vi "Checkers PvP.vi"() -> ()   [LabVIEW 2016]
uses:
  <vilib>/Utility/miscctls.llb/LVPositionTypeDef.ctl
  Game Info Global Variable.vi
  Board Layout Global Variable.vi
panel:
  out "P2 Bottom Right Marker":picture
  out "P2 Bottom Left Marker":picture
  out "P2 Top Left Marker":picture
  out "P2 Top Right Marker":picture
  out "P1 Bottom Left Marker":picture
  out "P1 Bottom Right Marker":picture
  out "P1 Top Right Marker":picture
  out "P1 Top Left Marker":picture
  in  "Save and Quit":bool
  out "Player 2 Name":string="Player 2"
  out "Player 1 Name":string="Player 1"
  out "P2 King 12":picture
  out "P2 King 11":picture
  out "P2 King 10":picture
  out "P2 King 9":picture
  out "P2 King 8":picture
  out "P2 King 7":picture
  out "P2 King 6":picture
  out "P2 King 5":picture
  out "P2 King 4":picture
  out "P2 King 3":picture
  out "P2 King 2":picture
  out "P2 King":picture
  out "P1 King 12":picture
  out "P1 King 11":picture
  out "P1 King 10":picture
  out "P1 King 9":picture
  out "P1 King 8":picture
  out "P1 King 7":picture
  out "P1 King 6":picture
  out "P1 King 5":picture
  out "P1 King 4":picture
  out "P1 King 3":picture
  out "P1 King 2":picture
  out "P1 King":picture
  out "P2 Piece Icon":picture
  out "P1 Piece Icon":picture
  out "P2 Piece 12":picture
  out "P2 Piece 11":picture
  out "P2 Piece 10":picture
  out "P2 Piece 9":picture
  out "P2 Piece 8":picture
  out "P2 Piece 7":picture
  out "P2 Piece 6":picture
  out "P2 Piece 5":picture
  out "P2 Piece 4":picture
  out "P2 Piece 3":picture
  out "P2 Piece 2":picture
  out "P1 Piece 12":picture caption="P1 Piece"
  out "P1 Piece 11":picture caption="P1 Piece"
  out "P1 Piece 10":picture caption="P1 Piece"
  out "P1 Piece 9":picture caption="P1 Piece"
  out "P1 Piece 8":picture caption="P1 Piece"
  out "P1 Piece 7":picture caption="P1 Piece"
  out "P1 Piece 6":picture caption="P1 Piece"
  out "P1 Piece 5":picture caption="P1 Piece"
  out "P1 Piece 4":picture caption="P1 Piece"
  out "P1 Piece 3":picture caption="P1 Piece"
  out "P2 Piece":picture
  out "P1 Piece 2":picture caption="P1 Piece"
  in  "TURN":bool
  out "Game String":string
  out "P2 Turn Light":bool
  out "P1 Turn Light":bool=TRUE
  out "P1 Piece":picture
  in  "stop":bool
  in  "Offer Draw":bool
  in  "Surrender":bool
  out "Player 2 Label":string="Player 1"
  out "Player 1 Label":string="Player 1"
  in  "Save":bool
  in  "Quit":bool
  # "Your Turn!"
  # "Your Turn!"
  # "678, \n56"
  # "764, \n56"
  # "512, \n56"
  # "594, \n56"
  # "637, \n99"
  # "469, \n99"
  # "553, \n99"
  # "720, \n99"
  # "355, \n141"
  # "400, \n141"
  # "512, \n140"
  # "594, \n140"
  # "678, \n140"
  # "828, \n141"
  # "873, \n141"
  # "764, \n140"
  # "828, \n184"
  # "873, \n184"
  # "355, \n184"
  # "400, \n184"
  # "469, \n183"
  # "553, \n183"
  # "637, \n183"
  # "720, \n183"
  # "355, \n225"
  # "828, \n225"
  # "873, \n225"
  # "400, \n225"
  # "764, \n224"
  # "512, \n224"
  # "595, \n224"
  # "678, \n224"
  # "828, \n267"
  # "873, \n267"
  # "355, \n267"
  # "400, \n267"
  # "469, \n266"
  # "553, \n266"
  # "720, \n266"
  # "637, \n266"
  # "355, \n309"
  # "828, \n309"
  # "400, \n309"
  # "873, \n309"
  # "678, \n308"
  # "764, \n308"
  # "512, \n308"
  # "595, \n308"
  # "355, \n351"
  # "400, \n351"
  # "873, \n351"
  # "828, \n351"
  # "553, \n350"
  # "637, \n350"
  # "720, \n350"
  # "469,\n350"
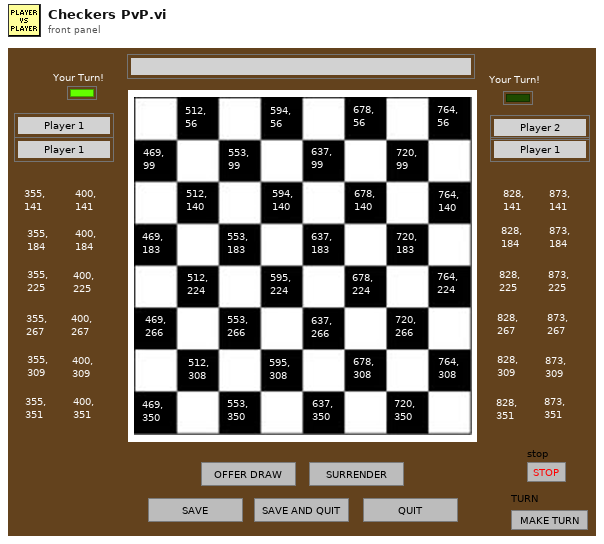
[diagram p1: front panel]
types:
  T1 = typedef "LVPositionTypeDef.ctl" = cluster{"Left":i32, "Top":i32}
  T2 = enum16{"Left Button", "Center Button", "Right Button", "Window Close"}
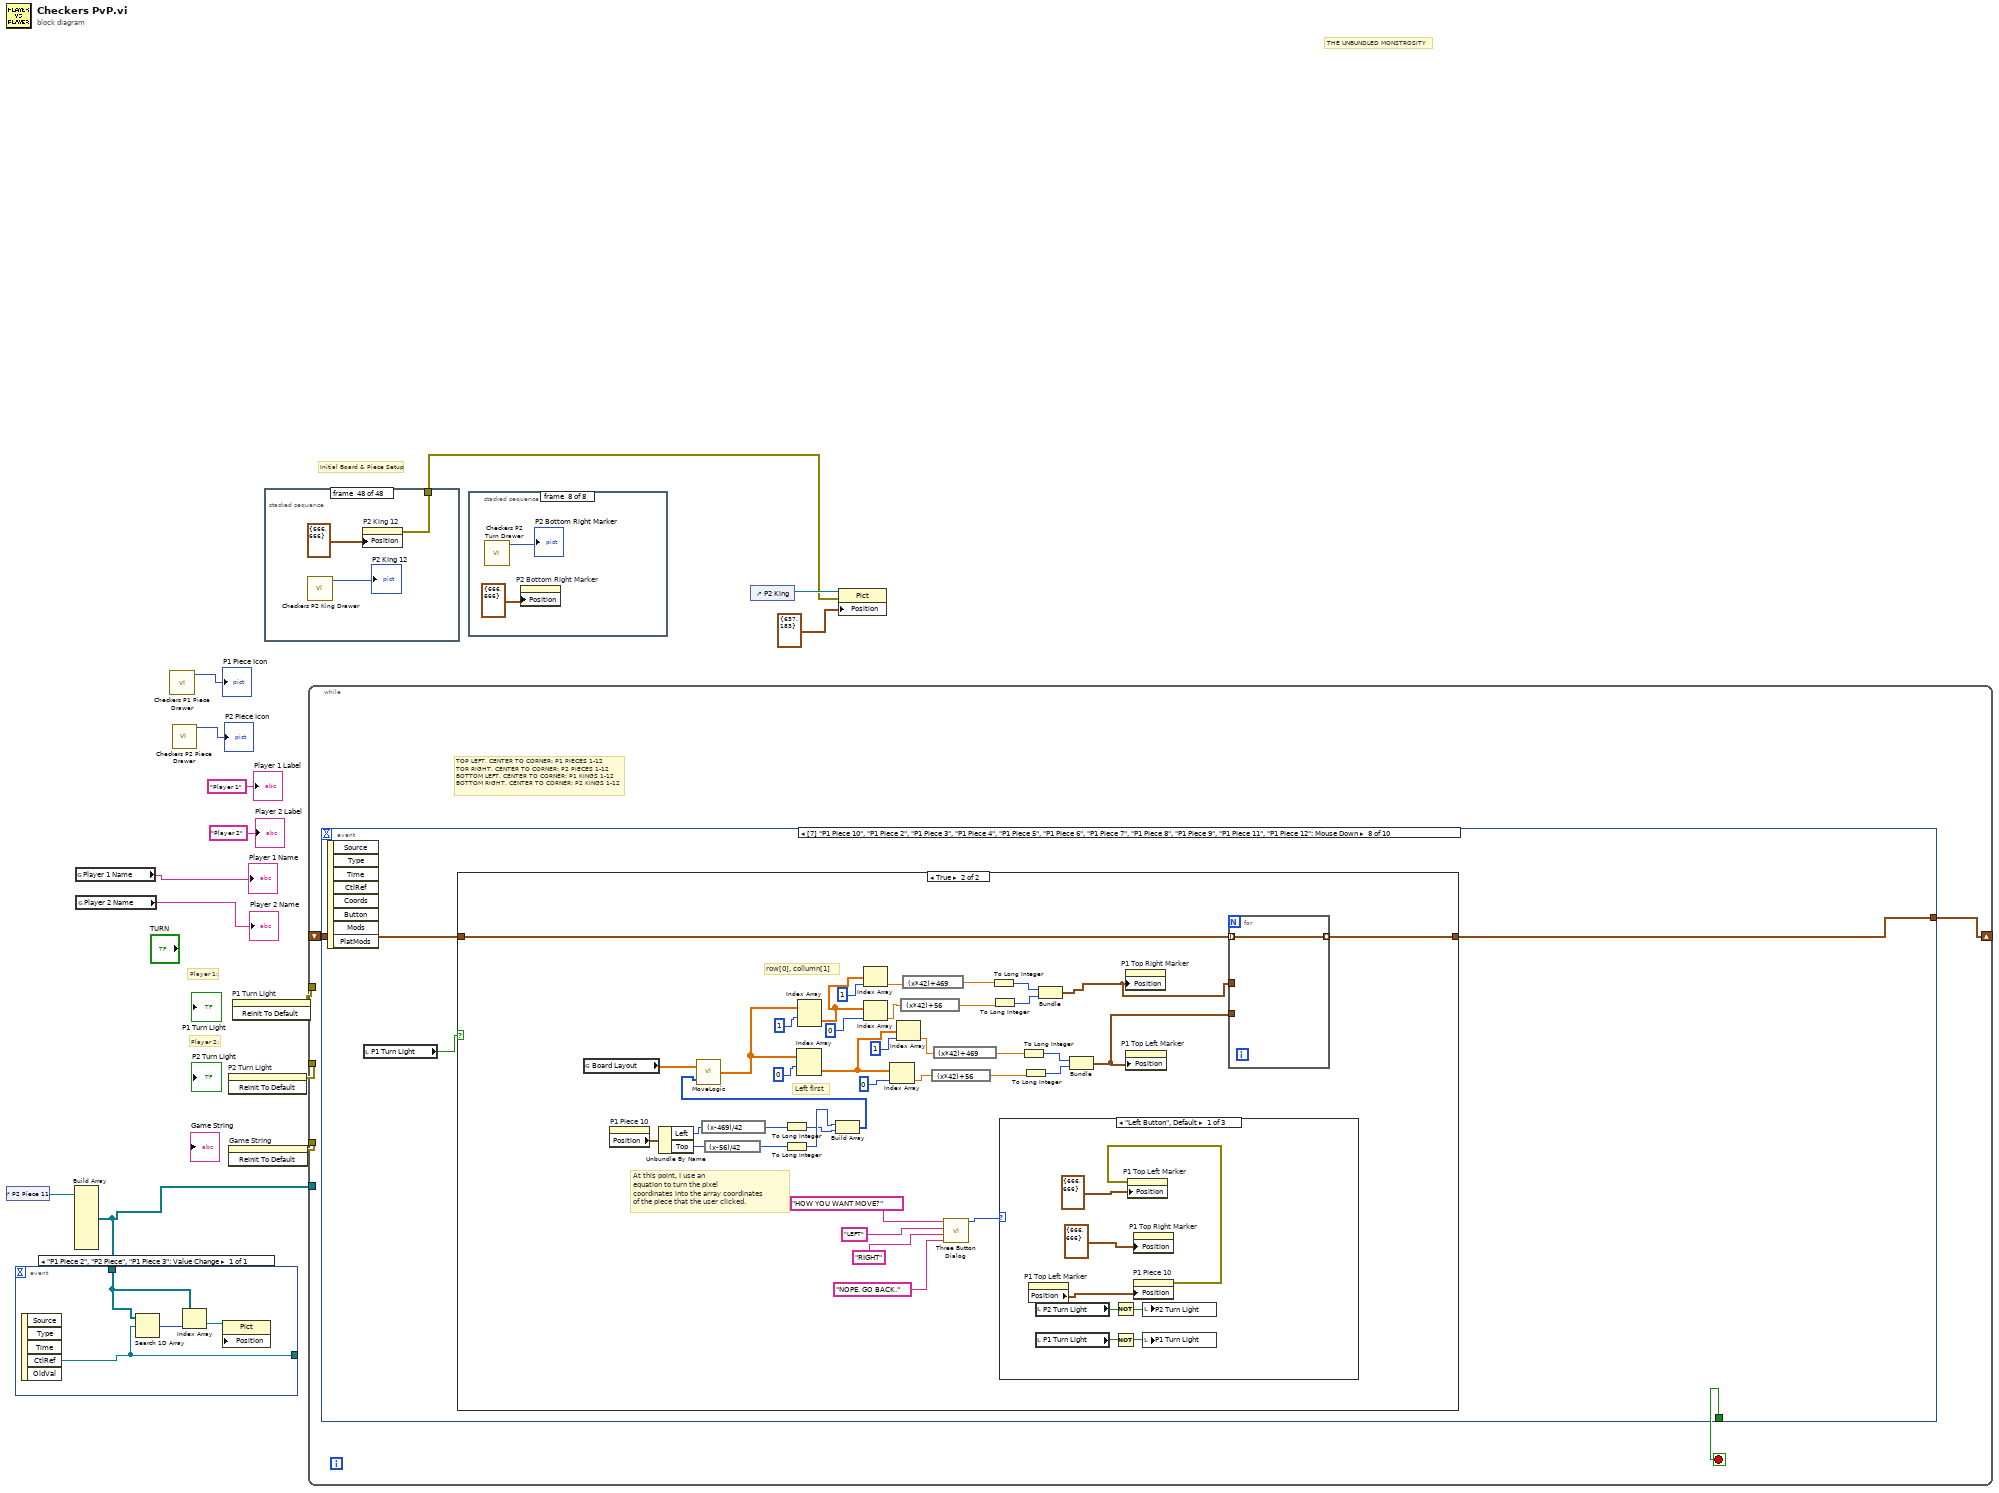
[diagram p0: block diagram]
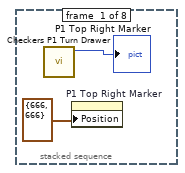
[diagram p2: hidden frame]
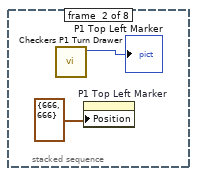
[diagram p3: hidden frame]
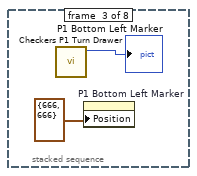
[diagram p4: hidden frame]
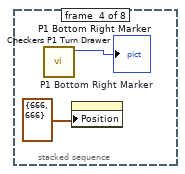
[diagram p5: hidden frame]
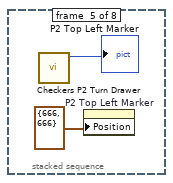
[diagram p6: hidden frame]
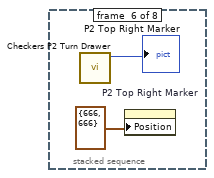
[diagram p7: hidden frame]
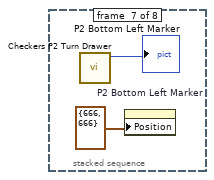
[diagram p8: hidden frame]
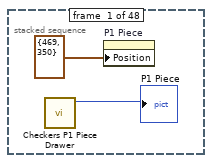
[diagram p9: hidden frame]
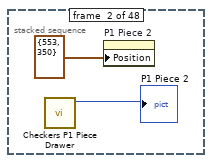
[diagram p10: hidden frame]
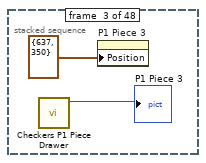
[diagram p11: hidden frame]
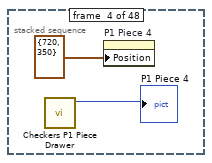
[diagram p12: hidden frame]
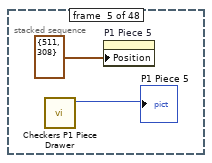
[diagram p13: hidden frame]
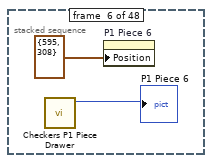
[diagram p14: hidden frame]
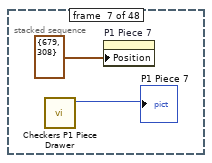
[diagram p15: hidden frame]
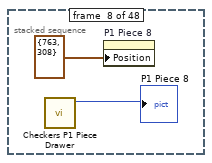
[diagram p16: hidden frame]
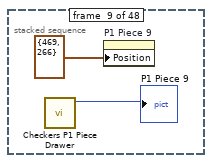
[diagram p17: hidden frame]
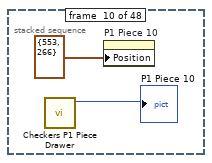
[diagram p18: hidden frame]
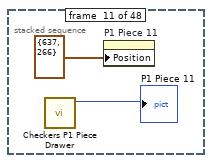
[diagram p19: hidden frame]
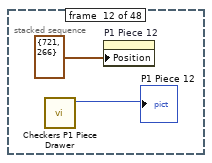
[diagram p20: hidden frame]
diagram:
  # "THE UNBUNDLED MONSTROSITY"
  # "Initial Board & Piece Setup"
  # "Player 2:"
  # "Player 1:"
  n1 = control-ref of="P2 Piece 11"() -> (w2:refnum<vi>)
  n2 = Build Array(w2) -> (w1:refnum<vi>[])  [unwired: 9 in]
  n3 = event shown="[0] \"P1 Piece 2\", \"P2 Piece\", \"P1 Piece 3\": Value Change" {
    selector: _ -> [_]
    dyn-events: _ -> [_]
    timeout: _ -> [_]
    tunnel: [w18] -> _
    tunnel: w1 -> [w17]
    event "P1 Piece 2", "P2 Piece", "P1 Piece 3": Value Change {
      n4 = event-data() -> ("CtlRef"=w18:refnum<vi>)  [unwired: 1 in, 4 out]
      n5 = Search 1D Array(1D array=w17, element=w18) -> (index of element=w16:i32)  [unwired: 1 in]
      n6 = Index Array(array=w17, index=w16) -> (element=w15:refnum<vi>)
      n7 = property class="Pict" props=["Position"](reference=w15) -> ()  [unwired: 2 in, 2 out]
    }
  }
  n8 = global read "Game Info Global Variable.vi" "Player 1 Name"() -> (→"Player 1 Name":string)
  n9 = global read "Game Info Global Variable.vi" "Player 2 Name"() -> (→"Player 2 Name":string)
  n10 = call "Checkers P1 Piece Drawer.vi"() -> ("new picture"=→"P1 Piece Icon":picture)  [unwired: 11 in]
  n11 = call "Checkers P2 Piece Drawer.vi"() -> ("new picture"=→"P2 Piece Icon":picture)  [unwired: 11 in]
  n12 = invoke on="P2 Turn Light" class="Bool (strict)" method="Reinit To Default"() -> (error out=w11:errorcluster)  [unwired: 3 in, 2 out]
  n13 = invoke on="Game String" class="Str" method="Reinit To Default"() -> (error out=w9:errorcluster)  [unwired: 3 in, 2 out]
  n14 = invoke on="P1 Turn Light" class="Bool (strict)" method="Reinit To Default"() -> (error out=w10:errorcluster)  [unwired: 3 in, 2 out]
  n15 = stacked-sequence {
    tunnel: [_ _ _ _ _ _ _ _ _ _ _ _ _ _ _ _ _ _ _ _ _ _ _ _ _ _ _ _ _ _ _ _ _ _ _ _ _ _ _ _ _ _ _ _ _ _ _ w113] -> w3
    frame #0 {
      n16 = call "Checkers P1 Piece Drawer.vi"() -> ("new picture"=→"P1 Piece":picture)  [unwired: 11 in]
      n17 = property on="P1 Piece" class="Pict"("Position"=T1 {"Left"=469, "Top"=350}) -> ()  [unwired: 2 in, 2 out]
    }
    frame #1 {
      n18 = call "Checkers P1 Piece Drawer.vi"() -> ("new picture"=→"P1 Piece 2":picture)  [unwired: 11 in]
      n19 = property on="P1 Piece 2" class="Pict"("Position"=T1 {"Left"=553, "Top"=350}) -> ()  [unwired: 2 in, 2 out]
    }
    frame #2 {
      n20 = call "Checkers P1 Piece Drawer.vi"() -> ("new picture"=→"P1 Piece 3":picture)  [unwired: 11 in]
      n21 = property on="P1 Piece 3" class="Pict"("Position"=T1 {"Left"=637, "Top"=350}) -> ()  [unwired: 2 in, 2 out]
    }
    frame #3 {
      n22 = call "Checkers P1 Piece Drawer.vi"() -> ("new picture"=→"P1 Piece 4":picture)  [unwired: 11 in]
      n23 = property on="P1 Piece 4" class="Pict"("Position"=T1 {"Left"=720, "Top"=350}) -> ()  [unwired: 2 in, 2 out]
    }
    frame #4 {
      n24 = call "Checkers P1 Piece Drawer.vi"() -> ("new picture"=→"P1 Piece 5":picture)  [unwired: 11 in]
      n25 = property on="P1 Piece 5" class="Pict"("Position"=T1 {"Left"=511, "Top"=308}) -> ()  [unwired: 2 in, 2 out]
    }
    frame #5 {
      n26 = call "Checkers P1 Piece Drawer.vi"() -> ("new picture"=→"P1 Piece 6":picture)  [unwired: 11 in]
      n27 = property on="P1 Piece 6" class="Pict"("Position"=T1 {"Left"=595, "Top"=308}) -> ()  [unwired: 2 in, 2 out]
    }
    frame #6 {
      n28 = call "Checkers P1 Piece Drawer.vi"() -> ("new picture"=→"P1 Piece 7":picture)  [unwired: 11 in]
      n29 = property on="P1 Piece 7" class="Pict"("Position"=T1 {"Left"=679, "Top"=308}) -> ()  [unwired: 2 in, 2 out]
    }
    frame #7 {
      n30 = call "Checkers P1 Piece Drawer.vi"() -> ("new picture"=→"P1 Piece 8":picture)  [unwired: 11 in]
      n31 = property on="P1 Piece 8" class="Pict"("Position"=T1 {"Left"=763, "Top"=308}) -> ()  [unwired: 2 in, 2 out]
    }
    frame #8 {
      n32 = call "Checkers P1 Piece Drawer.vi"() -> ("new picture"=→"P1 Piece 9":picture)  [unwired: 11 in]
      n33 = property on="P1 Piece 9" class="Pict"("Position"=T1 {"Left"=469, "Top"=266}) -> ()  [unwired: 2 in, 2 out]
    }
    frame #9 {
      n34 = call "Checkers P1 Piece Drawer.vi"() -> ("new picture"=→"P1 Piece 10":picture)  [unwired: 11 in]
      n35 = property on="P1 Piece 10" class="Pict"("Position"=T1 {"Left"=553, "Top"=266}) -> ()  [unwired: 2 in, 2 out]
    }
    frame #10 {
      n36 = call "Checkers P1 Piece Drawer.vi"() -> ("new picture"=→"P1 Piece 11":picture)  [unwired: 11 in]
      n37 = property on="P1 Piece 11" class="Pict"("Position"=T1 {"Left"=637, "Top"=266}) -> ()  [unwired: 2 in, 2 out]
    }
    frame #11 {
      n38 = call "Checkers P1 Piece Drawer.vi"() -> ("new picture"=→"P1 Piece 12":picture)  [unwired: 11 in]
      n39 = property on="P1 Piece 12" class="Pict"("Position"=T1 {"Left"=721, "Top"=266}) -> ()  [unwired: 2 in, 2 out]
    }
    frame #12 {
      n40 = call "Checkers P2 Piece Drawer.vi"() -> ("new picture"=→"P2 Piece":picture)  [unwired: 11 in]
      n41 = property on="P2 Piece" class="Pict"("Position"=T1 {"Left"=511, "Top"=140}) -> ()  [unwired: 2 in, 2 out]
    }
    frame #13 {
      n42 = call "Checkers P2 Piece Drawer.vi"() -> ("new picture"=→"P2 Piece 2":picture)  [unwired: 11 in]
      n43 = property on="P2 Piece 2" class="Pict"("Position"=T1 {"Left"=595, "Top"=140}) -> ()  [unwired: 2 in, 2 out]
    }
    frame #14 {
      n44 = call "Checkers P2 Piece Drawer.vi"() -> ("new picture"=→"P2 Piece 3":picture)  [unwired: 11 in]
      n45 = property on="P2 Piece 3" class="Pict"("Position"=T1 {"Left"=679, "Top"=140}) -> ()  [unwired: 2 in, 2 out]
    }
    frame #15 {
      n46 = call "Checkers P2 Piece Drawer.vi"() -> ("new picture"=→"P2 Piece 4":picture)  [unwired: 11 in]
      n47 = property on="P2 Piece 4" class="Pict"("Position"=T1 {"Left"=763, "Top"=140}) -> ()  [unwired: 2 in, 2 out]
    }
    frame #16 {
      n48 = call "Checkers P2 Piece Drawer.vi"() -> ("new picture"=→"P2 Piece 5":picture)  [unwired: 11 in]
      n49 = property on="P2 Piece 5" class="Pict"("Position"=T1 {"Left"=469, "Top"=98}) -> ()  [unwired: 2 in, 2 out]
    }
    frame #17 {
      n50 = call "Checkers P2 Piece Drawer.vi"() -> ("new picture"=→"P2 Piece 6":picture)  [unwired: 11 in]
      n51 = property on="P2 Piece 6" class="Pict"("Position"=T1 {"Left"=553, "Top"=98}) -> ()  [unwired: 2 in, 2 out]
    }
    frame #18 {
      n52 = call "Checkers P2 Piece Drawer.vi"() -> ("new picture"=→"P2 Piece 7":picture)  [unwired: 11 in]
      n53 = property on="P2 Piece 7" class="Pict"("Position"=T1 {"Left"=637, "Top"=98}) -> ()  [unwired: 2 in, 2 out]
    }
    frame #19 {
      n54 = call "Checkers P2 Piece Drawer.vi"() -> ("new picture"=→"P2 Piece 8":picture)  [unwired: 11 in]
      n55 = property on="P2 Piece 8" class="Pict"("Position"=T1 {"Left"=721, "Top"=98}) -> ()  [unwired: 2 in, 2 out]
    }
    frame #20 {
      n56 = call "Checkers P2 Piece Drawer.vi"() -> ("new picture"=→"P2 Piece 9":picture)  [unwired: 11 in]
      n57 = property on="P2 Piece 9" class="Pict"("Position"=T1 {"Left"=511, "Top"=56}) -> ()  [unwired: 2 in, 2 out]
    }
    frame #21 {
      n58 = call "Checkers P2 Piece Drawer.vi"() -> ("new picture"=→"P2 Piece 10":picture)  [unwired: 11 in]
      n59 = property on="P2 Piece 10" class="Pict"("Position"=T1 {"Left"=595, "Top"=56}) -> ()  [unwired: 2 in, 2 out]
    }
    frame #22 {
      n60 = call "Checkers P2 Piece Drawer.vi"() -> ("new picture"=→"P2 Piece 11":picture)  [unwired: 11 in]
      n61 = property on="P2 Piece 11" class="Pict"("Position"=T1 {"Left"=679, "Top"=56}) -> ()  [unwired: 2 in, 2 out]
    }
    frame #23 {
      n62 = call "Checkers P2 Piece Drawer.vi"() -> ("new picture"=→"P2 Piece 12":picture)  [unwired: 11 in]
      n63 = property on="P2 Piece 12" class="Pict"("Position"=T1 {"Left"=763, "Top"=56}) -> ()  [unwired: 2 in, 2 out]
    }
    frame #24 {
      n64 = call "Checkers P1 King Drawer.vi"() -> ("new picture"=→"P1 King":picture)  [unwired: 11 in]
      n65 = property on="P1 King" class="Pict"("Position"=T1 {"Left"=666, "Top"=666}) -> ()  [unwired: 2 in, 2 out]
    }
    frame #25 {
      n66 = call "Checkers P1 King Drawer.vi"() -> ("new picture"=→"P1 King 2":picture)  [unwired: 11 in]
      n67 = property on="P1 King 2" class="Pict"("Position"=T1 {"Left"=666, "Top"=666}) -> ()  [unwired: 2 in, 2 out]
    }
    frame #26 {
      n68 = call "Checkers P1 King Drawer.vi"() -> ("new picture"=→"P1 King 3":picture)  [unwired: 11 in]
      n69 = property on="P1 King 3" class="Pict"("Position"=T1 {"Left"=666, "Top"=666}) -> ()  [unwired: 2 in, 2 out]
    }
    frame #27 {
      n70 = call "Checkers P1 King Drawer.vi"() -> ("new picture"=→"P1 King 4":picture)  [unwired: 11 in]
      n71 = property on="P1 King 4" class="Pict"("Position"=T1 {"Left"=666, "Top"=666}) -> ()  [unwired: 2 in, 2 out]
    }
    frame #28 {
      n72 = call "Checkers P1 King Drawer.vi"() -> ("new picture"=→"P1 King 5":picture)  [unwired: 11 in]
      n73 = property on="P1 King 5" class="Pict"("Position"=T1 {"Left"=666, "Top"=666}) -> ()  [unwired: 2 in, 2 out]
    }
    frame #29 {
      n74 = call "Checkers P1 King Drawer.vi"() -> ("new picture"=→"P1 King 6":picture)  [unwired: 11 in]
      n75 = property on="P1 King 6" class="Pict"("Position"=T1 {"Left"=666, "Top"=666}) -> ()  [unwired: 2 in, 2 out]
    }
    frame #30 {
      n76 = call "Checkers P1 King Drawer.vi"() -> ("new picture"=→"P1 King 7":picture)  [unwired: 11 in]
      n77 = property on="P1 King 7" class="Pict"("Position"=T1 {"Left"=666, "Top"=666}) -> ()  [unwired: 2 in, 2 out]
    }
    frame #31 {
      n78 = call "Checkers P1 King Drawer.vi"() -> ("new picture"=→"P1 King 8":picture)  [unwired: 11 in]
      n79 = property on="P1 King 8" class="Pict"("Position"=T1 {"Left"=666, "Top"=666}) -> ()  [unwired: 2 in, 2 out]
    }
    frame #32 {
      n80 = call "Checkers P1 King Drawer.vi"() -> ("new picture"=→"P1 King 9":picture)  [unwired: 11 in]
      n81 = property on="P1 King 9" class="Pict"("Position"=T1 {"Left"=666, "Top"=666}) -> ()  [unwired: 2 in, 2 out]
    }
    frame #33 {
      n82 = call "Checkers P1 King Drawer.vi"() -> ("new picture"=→"P1 King 10":picture)  [unwired: 11 in]
      n83 = property on="P1 King 10" class="Pict"("Position"=T1 {"Left"=666, "Top"=666}) -> ()  [unwired: 2 in, 2 out]
    }
    frame #34 {
      n84 = call "Checkers P1 King Drawer.vi"() -> ("new picture"=→"P1 King 11":picture)  [unwired: 11 in]
      n85 = property on="P1 King 11" class="Pict"("Position"=T1 {"Left"=666, "Top"=666}) -> ()  [unwired: 2 in, 2 out]
    }
    frame #35 {
      n86 = call "Checkers P1 King Drawer.vi"() -> ("new picture"=→"P1 King 12":picture)  [unwired: 11 in]
      n87 = property on="P1 King 12" class="Pict"("Position"=T1 {"Left"=666, "Top"=666}) -> ()  [unwired: 2 in, 2 out]
    }
    frame #36 {
      n88 = call "Checkers P2 King Drawer.vi"() -> ("new picture"=→"P2 King":picture)  [unwired: 11 in]
      n89 = property on="P2 King" class="Pict"("Position"=T1 {"Left"=666, "Top"=666}) -> ()  [unwired: 2 in, 2 out]
    }
    frame #37 {
      n90 = call "Checkers P2 King Drawer.vi"() -> ("new picture"=→"P2 King 2":picture)  [unwired: 11 in]
      n91 = property on="P2 King 2" class="Pict"("Position"=T1 {"Left"=666, "Top"=666}) -> ()  [unwired: 2 in, 2 out]
    }
    frame #38 {
      n92 = call "Checkers P2 King Drawer.vi"() -> ("new picture"=→"P2 King 3":picture)  [unwired: 11 in]
      n93 = property on="P2 King 3" class="Pict"("Position"=T1 {"Left"=666, "Top"=666}) -> ()  [unwired: 2 in, 2 out]
    }
    frame #39 {
      n94 = call "Checkers P2 King Drawer.vi"() -> ("new picture"=→"P2 King 4":picture)  [unwired: 11 in]
      n95 = property on="P2 King 4" class="Pict"("Position"=T1 {"Left"=666, "Top"=666}) -> ()  [unwired: 2 in, 2 out]
    }
    frame #40 {
      n96 = call "Checkers P2 King Drawer.vi"() -> ("new picture"=→"P2 King 5":picture)  [unwired: 11 in]
      n97 = property on="P2 King 5" class="Pict"("Position"=T1 {"Left"=666, "Top"=666}) -> ()  [unwired: 2 in, 2 out]
    }
    frame #41 {
      n98 = call "Checkers P2 King Drawer.vi"() -> ("new picture"=→"P2 King 6":picture)  [unwired: 11 in]
      n99 = property on="P2 King 6" class="Pict"("Position"=T1 {"Left"=666, "Top"=666}) -> ()  [unwired: 2 in, 2 out]
    }
    frame #42 {
      n100 = call "Checkers P2 King Drawer.vi"() -> ("new picture"=→"P2 King 7":picture)  [unwired: 11 in]
      n101 = property on="P2 King 7" class="Pict"("Position"=T1 {"Left"=666, "Top"=666}) -> ()  [unwired: 2 in, 2 out]
    }
    frame #43 {
      n102 = call "Checkers P2 King Drawer.vi"() -> ("new picture"=→"P2 King 8":picture)  [unwired: 11 in]
      n103 = property on="P2 King 8" class="Pict"("Position"=T1 {"Left"=666, "Top"=666}) -> ()  [unwired: 2 in, 2 out]
    }
    frame #44 {
      n104 = call "Checkers P2 King Drawer.vi"() -> ("new picture"=→"P2 King 9":picture)  [unwired: 11 in]
      n105 = property on="P2 King 9" class="Pict"("Position"=T1 {"Left"=666, "Top"=666}) -> ()  [unwired: 2 in, 2 out]
    }
    frame #45 {
      n106 = call "Checkers P2 King Drawer.vi"() -> ("new picture"=→"P2 King 10":picture)  [unwired: 11 in]
      n107 = property on="P2 King 10" class="Pict"("Position"=T1 {"Left"=666, "Top"=666}) -> ()  [unwired: 2 in, 2 out]
    }
    frame #46 {
      n108 = call "Checkers P2 King Drawer.vi"() -> ("new picture"=→"P2 King 11":picture)  [unwired: 11 in]
      n109 = property on="P2 King 11" class="Pict"("Position"=T1 {"Left"=666, "Top"=666}) -> ()  [unwired: 2 in, 2 out]
    }
    frame #47 {
      n110 = call "Checkers P2 King Drawer.vi"() -> ("new picture"=→"P2 King 12":picture)  [unwired: 11 in]
      n111 = property on="P2 King 12" class="Pict"("Position"=T1 {"Left"=666, "Top"=666}) -> (error out=w113:errorcluster)  [unwired: 2 in, 1 out]
    }
  }
  n112 = while {
    tunnel: w11 -> [_]
    tunnel: w10 -> [_]
    tunnel: w9 -> [_]
    shift-right: [w117] -> _
    shift-left: _ -> [w116]
    tunnel: w1 -> [_]
    stop <- w118 stop-if-true
    # "TOP LEFT, CENTER TO CORNER: P1 PIECES 1-12\nTOR RIGHT, CENTER TO CORNER: P2 PIECES 1-12\nBOTTOM LEFT, CENTER TO CORNER: P1 KINGS 1-12\nBOTTOM RIGHT, CENTER TO CORNER: P2 KINGS 1-12"
    n113 = event shown="[7] \"P1 Piece 10\", \"P1 Piece 2\", \"P1 Piece 3\", \"P1 Piece 4\", \"P1 Piece 5\", \"P1 Piece 6\", \"P1 Piece 7\", \"P1 Piece 8\", \"P1 Piece 9\", \"P1 Piece 11\", \"P1 Piece 12\": Mouse Down" {
      selector: _ -> [_ _ _ _ _ _ _ _ _ _]
      dyn-events: _ -> [_ _ _ _ _ _ _ _ _ _]
      timeout: _ -> [_ _ _ _ _ _ _ _ _ _]
      tunnel: [_ "stop" _ _ _ _ _ _ _ _] -> w118
      tunnel: [w119 w120 w122 w172 w224 w347 w481 w496 w557 w658] -> w117
      tunnel: w116 -> [w119 w120 w122 w172 _ _ w481 w497 w557 w658]
      event Timeout {
        n114 = event-data() -> ()  [unwired: 1 in, 3 out]
      }
      event "stop": Value Change {
        n115 = event-data() -> ()  [unwired: 1 in, 6 out]
      }
      event "Offer Draw": Value Change {
        n116 = event-data() -> ()  [unwired: 1 in, 6 out]
        n117 = local read "P1 Turn Light"() -> (w123:bool)
        n118 = case shown="False" w123 {
          frame False {
            n119 = local read "Player 2 Name"() -> (w127:string)
            n120 = Format Into String(format string="%s offers a stalemate. Do you accept?", w127) -> (resulting string=w125:string)  [unwired: 2 in, 1 out]
            n121 = Two Button Dialog(message=w125, 1:"Decline" ("F button name (\"Cancel\")"), 2:"Accept" ("T button name (\"OK\")")) -> (T button?=w124:bool)
            n122 = case shown="True" w124 {
              frame False {
                # "Stalemate offer rejected. Do nothing."
              }
              frame True {
                w130 = "GAME OVER. It's a draw." ("format string")
                n123 = local write "Game String"(w130) -> ()
                n124 = Two Button Dialog(message=w130, 1:"Main Menu" ("F button name (\"Cancel\")"), 2:"New Game" ("T button name (\"OK\")")) -> (T button?=w133:bool)
                n125 = case shown="False" w133 {
                  frame False {
                    n126 = vi-ref "Checkers Main Menu.vi"() -> (w140:refnum<vi>)
                    n127 = invoke class="VI" method="Run VI"(reference=w140, "Wait until done"=FALSE ("Wait Until Done")) -> (reference out=w139:refnum<vi>, error out=w138:errorcluster)  [unwired: 3 in, 3 out]
                    n128 = invoke class="VI" method="FP.Open"(reference=w139, error in=w138, "Activate"=TRUE ("Activate?")) -> (error out=w137:errorcluster)  [unwired: 2 in, 4 out]
                    n129 = vi-ref "Checkers PvP.vi"() -> (w136:refnum<vi>)
                    n130 = invoke class="VI" method="Abort VI"(reference=w136, error in=w137) -> ()  [unwired: 1 in, 3 out]
                  }
                  frame True {
                    n131 = vi-ref "Checkers New Game.vi"() -> (w147:refnum<vi>)
                    n132 = invoke class="VI" method="Run VI"(reference=w147, "Wait until done"=FALSE ("Wait Until Done")) -> (reference out=w146:refnum<vi>, error out=w145:errorcluster)  [unwired: 3 in, 3 out]
                    n133 = invoke class="VI" method="FP.Open"(reference=w146, error in=w145, "Activate"=TRUE ("Activate?")) -> (error out=w144:errorcluster)  [unwired: 2 in, 4 out]
                    n134 = vi-ref "Checkers PvP.vi"() -> (w143:refnum<vi>)
                    n135 = invoke class="VI" method="Abort VI"(reference=w143, error in=w144) -> ()  [unwired: 1 in, 3 out]
                  }
                }
              }
            }
          }
          frame True {
            n136 = local read "Player 1 Name"() -> (w151:string)
            n137 = Format Into String(format string="%s offers a stalemate. Do you accept?", w151) -> (resulting string=w149:string)  [unwired: 2 in, 1 out]
            n138 = Two Button Dialog(message=w149, 1:"Decline" ("F button name (\"Cancel\")"), 2:"Accept" ("T button name (\"OK\")")) -> (T button?=w148:bool)
            n139 = case shown="True" w148 {
              frame False {
                # "Stalemate offer was rejected. Do nothing."
              }
              frame True {
                w154 = "GAME OVER. Stalemate." ("format string")
                n140 = local write "Game String"(w154) -> ()
                n141 = Two Button Dialog(message=w154, 1:"Main Menu" ("F button name (\"Cancel\")"), 2:"New Game" ("T button name (\"OK\")")) -> (T button?=w157:bool)
                n142 = case shown="False" w157 {
                  frame False {
                    n143 = vi-ref "Checkers Main Menu.vi"() -> (w164:refnum<vi>)
                    n144 = invoke class="VI" method="Run VI"(reference=w164, "Wait until done"=FALSE ("Wait Until Done")) -> (reference out=w163:refnum<vi>, error out=w162:errorcluster)  [unwired: 3 in, 3 out]
                    n145 = invoke class="VI" method="FP.Open"(reference=w163, error in=w162, "Activate"=TRUE ("Activate?")) -> (error out=w161:errorcluster)  [unwired: 2 in, 4 out]
                    n146 = vi-ref "Checkers PvP.vi"() -> (w160:refnum<vi>)
                    n147 = invoke class="VI" method="Abort VI"(reference=w160, error in=w161) -> ()  [unwired: 1 in, 3 out]
                  }
                  frame True {
                    n148 = vi-ref "Checkers New Game.vi"() -> (w171:refnum<vi>)
                    n149 = invoke class="VI" method="Run VI"(reference=w171, "Wait until done"=FALSE ("Wait Until Done")) -> (reference out=w170:refnum<vi>, error out=w169:errorcluster)  [unwired: 3 in, 3 out]
                    n150 = invoke class="VI" method="FP.Open"(reference=w170, error in=w169, "Activate"=TRUE ("Activate?")) -> (error out=w168:errorcluster)  [unwired: 2 in, 4 out]
                    n151 = vi-ref "Checkers PvP.vi"() -> (w167:refnum<vi>)
                    n152 = invoke class="VI" method="Abort VI"(reference=w167, error in=w168) -> ()  [unwired: 1 in, 3 out]
                  }
                }
              }
            }
          }
        }
      }
      event "Surrender": Value Change {
        n153 = event-data() -> ()  [unwired: 1 in, 6 out]
        n154 = Two Button Dialog(message="Are you sure you want to surrender?", 1:"No" ("F button name (\"Cancel\")"), 2:"Yes" ("T button name (\"OK\")")) -> (T button?=w173:bool)
        n155 = case shown="True" w173 {
          frame False {
            # "Player changed mind, didn't surrender. Do nothing."
          }
          frame True {
            n156 = local read "P1 Turn Light"() -> (w177:bool)
            n157 = case shown="True" w177 {
              frame False {
                n158 = local read "Player 1 Name"() -> (w178:string)
                n159 = Format Into String(format string="GAME OVER. %s WINS!", w178) -> (resulting string=w182:string)  [unwired: 2 in, 1 out]
                n160 = local write "Game String"(w182) -> ()
                n161 = Two Button Dialog(message=w182, 1:"Main Menu" ("F button name (\"Cancel\")"), 2:"New Game" ("T button name (\"OK\")")) -> (T button?=w179:bool)
                n162 = case shown="True" w179 {
                  frame False {
                    n163 = vi-ref "Checkers Main Menu.vi"() -> (w190:refnum<vi>)
                    n164 = invoke class="VI" method="Run VI"(reference=w190, "Wait until done"=FALSE ("Wait Until Done")) -> (reference out=w189:refnum<vi>, error out=w188:errorcluster)  [unwired: 3 in, 3 out]
                    n165 = invoke class="VI" method="FP.Open"(reference=w189, error in=w188, "Activate"=TRUE ("Activate?")) -> (error out=w187:errorcluster)  [unwired: 2 in, 4 out]
                    n166 = vi-ref "Checkers PvP.vi"() -> (w186:refnum<vi>)
                    n167 = invoke class="VI" method="Abort VI"(reference=w186, error in=w187) -> ()  [unwired: 1 in, 3 out]
                  }
                  frame True {
                    n168 = vi-ref "Checkers New Game.vi"() -> (w200:refnum<vi>)
                    n169 = vi-ref "Checkers Gymnopedie Music Player.vi"() -> (w191:refnum<vi>)
                    n170 = invoke class="VI" method="Run VI"(reference=w191, "Wait until done"=FALSE ("Wait Until Done")) -> ()  [unwired: 3 in, 5 out]
                    n171 = invoke class="VI" method="Run VI"(reference=w200, "Wait until done"=FALSE ("Wait Until Done")) -> (reference out=w199:refnum<vi>, error out=w198:errorcluster)  [unwired: 3 in, 3 out]
                    n172 = vi-ref "Checkers Palladio Music Player.vi"() -> (w193:refnum<vi>)
                    n173 = invoke class="VI" method="FP.Open"(reference=w199, error in=w198, "Activate"=TRUE ("Activate?")) -> (error out=w197:errorcluster)  [unwired: 2 in, 4 out]
                    n174 = vi-ref "Checkers PvP.vi"() -> (w196:refnum<vi>)
                    n175 = invoke class="VI" method="Abort VI"(reference=w193) -> ()  [unwired: 2 in, 3 out]
                    n176 = invoke class="VI" method="Abort VI"(reference=w196, error in=w197) -> ()  [unwired: 1 in, 3 out]
                  }
                }
              }
              frame True {
                n177 = local read "Player 2 Name"() -> (w201:string)
                n178 = Format Into String(format string="GAME OVER. %s WINS!", w201) -> (resulting string=w205:string)  [unwired: 2 in, 1 out]
                n179 = local write "Game String"(w205) -> ()
                n180 = Two Button Dialog(message=w205, 1:"Main Menu" ("F button name (\"Cancel\")"), 2:"New Game" ("T button name (\"OK\")")) -> (T button?=w202:bool)
                n181 = case shown="True" w202 {
                  frame False {
                    n182 = vi-ref "Checkers Main Menu.vi"() -> (w213:refnum<vi>)
                    n183 = invoke class="VI" method="Run VI"(reference=w213, "Wait until done"=FALSE ("Wait Until Done")) -> (reference out=w212:refnum<vi>, error out=w211:errorcluster)  [unwired: 3 in, 3 out]
                    n184 = invoke class="VI" method="FP.Open"(reference=w212, error in=w211, "Activate"=TRUE ("Activate?")) -> (error out=w210:errorcluster)  [unwired: 2 in, 4 out]
                    n185 = vi-ref "Checkers PvP.vi"() -> (w209:refnum<vi>)
                    n186 = invoke class="VI" method="Abort VI"(reference=w209, error in=w210) -> ()  [unwired: 1 in, 3 out]
                  }
                  frame True {
                    n187 = vi-ref "Checkers New Game.vi"() -> (w223:refnum<vi>)
                    n188 = vi-ref "Checkers Gymnopedie Music Player.vi"() -> (w214:refnum<vi>)
                    n189 = invoke class="VI" method="Run VI"(reference=w223, "Wait until done"=FALSE ("Wait Until Done")) -> (reference out=w222:refnum<vi>, error out=w221:errorcluster)  [unwired: 3 in, 3 out]
                    n190 = invoke class="VI" method="Run VI"(reference=w214, "Wait until done"=FALSE ("Wait Until Done")) -> ()  [unwired: 3 in, 5 out]
                    n191 = vi-ref "Checkers Palladio Music Player.vi"() -> (w216:refnum<vi>)
                    n192 = invoke class="VI" method="FP.Open"(reference=w222, error in=w221, "Activate"=TRUE ("Activate?")) -> (error out=w220:errorcluster)  [unwired: 2 in, 4 out]
                    n193 = vi-ref "Checkers PvP.vi"() -> (w219:refnum<vi>)
                    n194 = invoke class="VI" method="Abort VI"(reference=w216) -> ()  [unwired: 2 in, 3 out]
                    n195 = invoke class="VI" method="Abort VI"(reference=w219, error in=w220) -> ()  [unwired: 1 in, 3 out]
                  }
                }
              }
            }
          }
        }
      }
      event "Save": Value Change {
        n196 = event-data() -> ()  [unwired: 1 in, 6 out]
        n197 = global read "Game Info Global Variable.vi" "P1 King Text Green Color"() -> (w283:i32)
        n198 = global read "Game Info Global Variable.vi" "P2 King Text Green Color"() -> (w277:i32)
        n199 = global read "Game Info Global Variable.vi" "P1 King Text Blue Color"() -> (w282:i32)
        n200 = global read "Game Info Global Variable.vi" "P2 King Text Blue Color"() -> (w276:i32)
        n201 = global read "Game Info Global Variable.vi" "P1 King Text Red Color"() -> (w284:i32)
        n202 = global read "Game Info Global Variable.vi" "P2 King Text Red Color"() -> (w278:i32)
        n203 = global read "Game Info Global Variable.vi" "P1 Green Color"() -> (w286:i32)
        n204 = global read "Game Info Global Variable.vi" "P2 Green Color"() -> (w280:i32)
        n205 = local read "Player 1 Name"() -> (w290:string)
        n206 = local read "Player 2 Name"() -> (w289:string)
        n207 = global read "Game Info Global Variable.vi" "P1 Red Color"() -> (w287:i32)
        n208 = global read "Game Info Global Variable.vi" "P1 Blue Color"() -> (w285:i32)
        n209 = global read "Game Info Global Variable.vi" "P2 Blue Color"() -> (w279:i32)
        n210 = global read "Game Info Global Variable.vi" "P2 Red Color"() -> (w281:i32)
        n211 = Format Into String(w290, w289, w287, w286, w285, w284, w283, w282, w281, w280, w279, w278, w277, w276) -> (resulting string=w288:refnum<file>)  [unwired: 3 in, 1 out]
        n212 = stacked-sequence {
          tunnel: [w291 _ _ _ _ _ _ _ _ _ _ _ _ _ _ _ _ _ _ _ _ _ _ _ _ _ _ _ _ _ _ _ _ _ _ _ _ _ _ _ _ _ _ _ _ _ _ _] -> w275
          tunnel: [_ w292 _ _ _ _ _ _ _ _ _ _ _ _ _ _ _ _ _ _ _ _ _ _ _ _ _ _ _ _ _ _ _ _ _ _ _ _ _ _ _ _ _ _ _ _ _ _] -> w274
          tunnel: [_ _ w293 _ _ _ _ _ _ _ _ _ _ _ _ _ _ _ _ _ _ _ _ _ _ _ _ _ _ _ _ _ _ _ _ _ _ _ _ _ _ _ _ _ _ _ _ _] -> w273
          tunnel: [_ _ _ w294 _ _ _ _ _ _ _ _ _ _ _ _ _ _ _ _ _ _ _ _ _ _ _ _ _ _ _ _ _ _ _ _ _ _ _ _ _ _ _ _ _ _ _ _] -> w272
          tunnel: [_ _ _ _ w295 _ _ _ _ _ _ _ _ _ _ _ _ _ _ _ _ _ _ _ _ _ _ _ _ _ _ _ _ _ _ _ _ _ _ _ _ _ _ _ _ _ _ _] -> w271
          tunnel: [_ _ _ _ _ w296 _ _ _ _ _ _ _ _ _ _ _ _ _ _ _ _ _ _ _ _ _ _ _ _ _ _ _ _ _ _ _ _ _ _ _ _ _ _ _ _ _ _] -> w270
          tunnel: [_ _ _ _ _ _ w297 _ _ _ _ _ _ _ _ _ _ _ _ _ _ _ _ _ _ _ _ _ _ _ _ _ _ _ _ _ _ _ _ _ _ _ _ _ _ _ _ _] -> w269
          tunnel: [_ _ _ _ _ _ _ w298 _ _ _ _ _ _ _ _ _ _ _ _ _ _ _ _ _ _ _ _ _ _ _ _ _ _ _ _ _ _ _ _ _ _ _ _ _ _ _ _] -> w268
          tunnel: [_ _ _ _ _ _ _ _ w299 _ _ _ _ _ _ _ _ _ _ _ _ _ _ _ _ _ _ _ _ _ _ _ _ _ _ _ _ _ _ _ _ _ _ _ _ _ _ _] -> w267
          tunnel: [_ _ _ _ _ _ _ _ _ w300 _ _ _ _ _ _ _ _ _ _ _ _ _ _ _ _ _ _ _ _ _ _ _ _ _ _ _ _ _ _ _ _ _ _ _ _ _ _] -> w266
          tunnel: [_ _ _ _ _ _ _ _ _ _ w301 _ _ _ _ _ _ _ _ _ _ _ _ _ _ _ _ _ _ _ _ _ _ _ _ _ _ _ _ _ _ _ _ _ _ _ _ _] -> w265
          tunnel: [_ _ _ _ _ _ _ _ _ _ _ w302 _ _ _ _ _ _ _ _ _ _ _ _ _ _ _ _ _ _ _ _ _ _ _ _ _ _ _ _ _ _ _ _ _ _ _ _] -> w264
          tunnel: [_ _ _ _ _ _ _ _ _ _ _ _ w303 _ _ _ _ _ _ _ _ _ _ _ _ _ _ _ _ _ _ _ _ _ _ _ _ _ _ _ _ _ _ _ _ _ _ _] -> w262
          tunnel: [_ _ _ _ _ _ _ _ _ _ _ _ _ w304 _ _ _ _ _ _ _ _ _ _ _ _ _ _ _ _ _ _ _ _ _ _ _ _ _ _ _ _ _ _ _ _ _ _] -> w261
          tunnel: [_ _ _ _ _ _ _ _ _ _ _ _ _ _ w305 _ _ _ _ _ _ _ _ _ _ _ _ _ _ _ _ _ _ _ _ _ _ _ _ _ _ _ _ _ _ _ _ _] -> w260
          tunnel: [_ _ _ _ _ _ _ _ _ _ _ _ _ _ _ w306 _ _ _ _ _ _ _ _ _ _ _ _ _ _ _ _ _ _ _ _ _ _ _ _ _ _ _ _ _ _ _ _] -> w259
          tunnel: [_ _ _ _ _ _ _ _ _ _ _ _ _ _ _ _ w307 _ _ _ _ _ _ _ _ _ _ _ _ _ _ _ _ _ _ _ _ _ _ _ _ _ _ _ _ _ _ _] -> w258
          tunnel: [_ _ _ _ _ _ _ _ _ _ _ _ _ _ _ _ _ w308 _ _ _ _ _ _ _ _ _ _ _ _ _ _ _ _ _ _ _ _ _ _ _ _ _ _ _ _ _ _] -> w257
          tunnel: [_ _ _ _ _ _ _ _ _ _ _ _ _ _ _ _ _ _ w309 _ _ _ _ _ _ _ _ _ _ _ _ _ _ _ _ _ _ _ _ _ _ _ _ _ _ _ _ _] -> w256
          tunnel: [_ _ _ _ _ _ _ _ _ _ _ _ _ _ _ _ _ _ _ w310 _ _ _ _ _ _ _ _ _ _ _ _ _ _ _ _ _ _ _ _ _ _ _ _ _ _ _ _] -> w255
          tunnel: [_ _ _ _ _ _ _ _ _ _ _ _ _ _ _ _ _ _ _ _ w311 _ _ _ _ _ _ _ _ _ _ _ _ _ _ _ _ _ _ _ _ _ _ _ _ _ _ _] -> w254
          tunnel: [_ _ _ _ _ _ _ _ _ _ _ _ _ _ _ _ _ _ _ _ _ w312 _ _ _ _ _ _ _ _ _ _ _ _ _ _ _ _ _ _ _ _ _ _ _ _ _ _] -> w253
          tunnel: [_ _ _ _ _ _ _ _ _ _ _ _ _ _ _ _ _ _ _ _ _ _ w313 _ _ _ _ _ _ _ _ _ _ _ _ _ _ _ _ _ _ _ _ _ _ _ _ _] -> w252
          tunnel: [_ _ _ _ _ _ _ _ _ _ _ _ _ _ _ _ _ _ _ _ _ _ _ w314 _ _ _ _ _ _ _ _ _ _ _ _ _ _ _ _ _ _ _ _ _ _ _ _] -> w251
          tunnel: [_ _ _ _ _ _ _ _ _ _ _ _ _ _ _ _ _ _ _ _ _ _ _ _ w315 _ _ _ _ _ _ _ _ _ _ _ _ _ _ _ _ _ _ _ _ _ _ _] -> w249
          tunnel: [_ _ _ _ _ _ _ _ _ _ _ _ _ _ _ _ _ _ _ _ _ _ _ _ _ w316 _ _ _ _ _ _ _ _ _ _ _ _ _ _ _ _ _ _ _ _ _ _] -> w248
          tunnel: [_ _ _ _ _ _ _ _ _ _ _ _ _ _ _ _ _ _ _ _ _ _ _ _ _ _ w317 _ _ _ _ _ _ _ _ _ _ _ _ _ _ _ _ _ _ _ _ _] -> w247
          tunnel: [_ _ _ _ _ _ _ _ _ _ _ _ _ _ _ _ _ _ _ _ _ _ _ _ _ _ _ w318 _ _ _ _ _ _ _ _ _ _ _ _ _ _ _ _ _ _ _ _] -> w246
          tunnel: [_ _ _ _ _ _ _ _ _ _ _ _ _ _ _ _ _ _ _ _ _ _ _ _ _ _ _ _ w319 _ _ _ _ _ _ _ _ _ _ _ _ _ _ _ _ _ _ _] -> w245
          tunnel: [_ _ _ _ _ _ _ _ _ _ _ _ _ _ _ _ _ _ _ _ _ _ _ _ _ _ _ _ _ w320 _ _ _ _ _ _ _ _ _ _ _ _ _ _ _ _ _ _] -> w244
          tunnel: [_ _ _ _ _ _ _ _ _ _ _ _ _ _ _ _ _ _ _ _ _ _ _ _ _ _ _ _ _ _ w321 _ _ _ _ _ _ _ _ _ _ _ _ _ _ _ _ _] -> w243
          tunnel: [_ _ _ _ _ _ _ _ _ _ _ _ _ _ _ _ _ _ _ _ _ _ _ _ _ _ _ _ _ _ _ w322 _ _ _ _ _ _ _ _ _ _ _ _ _ _ _ _] -> w242
          tunnel: [_ _ _ _ _ _ _ _ _ _ _ _ _ _ _ _ _ _ _ _ _ _ _ _ _ _ _ _ _ _ _ _ w323 _ _ _ _ _ _ _ _ _ _ _ _ _ _ _] -> w241
          tunnel: [_ _ _ _ _ _ _ _ _ _ _ _ _ _ _ _ _ _ _ _ _ _ _ _ _ _ _ _ _ _ _ _ _ w324 _ _ _ _ _ _ _ _ _ _ _ _ _ _] -> w240
          tunnel: [_ _ _ _ _ _ _ _ _ _ _ _ _ _ _ _ _ _ _ _ _ _ _ _ _ _ _ _ _ _ _ _ _ _ w325 _ _ _ _ _ _ _ _ _ _ _ _ _] -> w239
          tunnel: [_ _ _ _ _ _ _ _ _ _ _ _ _ _ _ _ _ _ _ _ _ _ _ _ _ _ _ _ _ _ _ _ _ _ _ w326 _ _ _ _ _ _ _ _ _ _ _ _] -> w238
          tunnel: [_ _ _ _ _ _ _ _ _ _ _ _ _ _ _ _ _ _ _ _ _ _ _ _ _ _ _ _ _ _ _ _ _ _ _ _ w327 _ _ _ _ _ _ _ _ _ _ _] -> w236
          tunnel: [_ _ _ _ _ _ _ _ _ _ _ _ _ _ _ _ _ _ _ _ _ _ _ _ _ _ _ _ _ _ _ _ _ _ _ _ _ w328 _ _ _ _ _ _ _ _ _ _] -> w235
          tunnel: [_ _ _ _ _ _ _ _ _ _ _ _ _ _ _ _ _ _ _ _ _ _ _ _ _ _ _ _ _ _ _ _ _ _ _ _ _ _ w329 _ _ _ _ _ _ _ _ _] -> w234
          tunnel: [_ _ _ _ _ _ _ _ _ _ _ _ _ _ _ _ _ _ _ _ _ _ _ _ _ _ _ _ _ _ _ _ _ _ _ _ _ _ _ w330 _ _ _ _ _ _ _ _] -> w233
          tunnel: [_ _ _ _ _ _ _ _ _ _ _ _ _ _ _ _ _ _ _ _ _ _ _ _ _ _ _ _ _ _ _ _ _ _ _ _ _ _ _ _ w331 _ _ _ _ _ _ _] -> w232
          tunnel: [_ _ _ _ _ _ _ _ _ _ _ _ _ _ _ _ _ _ _ _ _ _ _ _ _ _ _ _ _ _ _ _ _ _ _ _ _ _ _ _ _ w332 _ _ _ _ _ _] -> w231
          tunnel: [_ _ _ _ _ _ _ _ _ _ _ _ _ _ _ _ _ _ _ _ _ _ _ _ _ _ _ _ _ _ _ _ _ _ _ _ _ _ _ _ _ _ w333 _ _ _ _ _] -> w230
          tunnel: [_ _ _ _ _ _ _ _ _ _ _ _ _ _ _ _ _ _ _ _ _ _ _ _ _ _ _ _ _ _ _ _ _ _ _ _ _ _ _ _ _ _ _ w334 _ _ _ _] -> w229
          tunnel: [_ _ _ _ _ _ _ _ _ _ _ _ _ _ _ _ _ _ _ _ _ _ _ _ _ _ _ _ _ _ _ _ _ _ _ _ _ _ _ _ _ _ _ _ w335 _ _ _] -> w228
          tunnel: [_ _ _ _ _ _ _ _ _ _ _ _ _ _ _ _ _ _ _ _ _ _ _ _ _ _ _ _ _ _ _ _ _ _ _ _ _ _ _ _ _ _ _ _ _ w336 _ _] -> w227
          tunnel: [_ _ _ _ _ _ _ _ _ _ _ _ _ _ _ _ _ _ _ _ _ _ _ _ _ _ _ _ _ _ _ _ _ _ _ _ _ _ _ _ _ _ _ _ _ _ w337 _] -> w226
          tunnel: [_ _ _ _ _ _ _ _ _ _ _ _ _ _ _ _ _ _ _ _ _ _ _ _ _ _ _ _ _ _ _ _ _ _ _ _ _ _ _ _ _ _ _ _ _ _ _ w338] -> w225
          frame #0 {
            n213 = property on="P1 Piece" class="Pict"() -> ("Position"=w291:T1)  [unwired: 2 in, 2 out]
          }
          frame #1 {
            n214 = property on="P1 Piece 2" class="Pict"() -> ("Position"=w292:T1)  [unwired: 2 in, 2 out]
          }
          frame #2 {
            n215 = property on="P1 Piece 3" class="Pict"() -> ("Position"=w293:T1)  [unwired: 2 in, 2 out]
          }
          frame #3 {
            n216 = property on="P1 Piece 4" class="Pict"() -> ("Position"=w294:T1)  [unwired: 2 in, 2 out]
          }
          frame #4 {
            n217 = property on="P1 Piece 5" class="Pict"() -> ("Position"=w295:T1)  [unwired: 2 in, 2 out]
          }
          frame #5 {
            n218 = property on="P1 Piece 6" class="Pict"() -> ("Position"=w296:T1)  [unwired: 2 in, 2 out]
          }
          frame #6 {
            n219 = property on="P1 Piece 7" class="Pict"() -> ("Position"=w297:T1)  [unwired: 2 in, 2 out]
          }
          frame #7 {
            n220 = property on="P1 Piece 8" class="Pict"() -> ("Position"=w298:T1)  [unwired: 2 in, 2 out]
          }
          frame #8 {
            n221 = property on="P1 Piece 9" class="Pict"() -> ("Position"=w299:T1)  [unwired: 2 in, 2 out]
          }
          frame #9 {
            n222 = property on="P1 Piece 10" class="Pict"() -> ("Position"=w300:T1)  [unwired: 2 in, 2 out]
          }
          frame #10 {
            n223 = property on="P1 Piece 11" class="Pict"() -> ("Position"=w301:T1)  [unwired: 2 in, 2 out]
          }
          frame #11 {
            n224 = property on="P1 Piece 12" class="Pict"() -> ("Position"=w302:T1)  [unwired: 2 in, 2 out]
          }
          frame #12 {
            n225 = property on="P2 Piece" class="Pict"() -> ("Position"=w303:T1)  [unwired: 2 in, 2 out]
          }
          frame #13 {
            n226 = property on="P2 Piece 2" class="Pict"() -> ("Position"=w304:T1)  [unwired: 2 in, 2 out]
          }
          frame #14 {
            n227 = property on="P2 Piece 3" class="Pict"() -> ("Position"=w305:T1)  [unwired: 2 in, 2 out]
          }
          frame #15 {
            n228 = property on="P2 Piece 4" class="Pict"() -> ("Position"=w306:T1)  [unwired: 2 in, 2 out]
          }
          frame #16 {
            n229 = property on="P2 Piece 5" class="Pict"() -> ("Position"=w307:T1)  [unwired: 2 in, 2 out]
          }
          frame #17 {
            n230 = property on="P2 Piece 6" class="Pict"() -> ("Position"=w308:T1)  [unwired: 2 in, 2 out]
          }
          frame #18 {
            n231 = property on="P2 Piece 7" class="Pict"() -> ("Position"=w309:T1)  [unwired: 2 in, 2 out]
          }
          frame #19 {
            n232 = property on="P2 Piece 8" class="Pict"() -> ("Position"=w310:T1)  [unwired: 2 in, 2 out]
          }
          frame #20 {
            n233 = property on="P2 Piece 9" class="Pict"() -> ("Position"=w311:T1)  [unwired: 2 in, 2 out]
          }
          frame #21 {
            n234 = property on="P2 Piece 10" class="Pict"() -> ("Position"=w312:T1)  [unwired: 2 in, 2 out]
          }
          frame #22 {
            n235 = property on="P2 Piece 11" class="Pict"() -> ("Position"=w313:T1)  [unwired: 2 in, 2 out]
          }
          frame #23 {
            n236 = property on="P2 Piece 12" class="Pict"() -> ("Position"=w314:T1)  [unwired: 2 in, 2 out]
          }
          frame #24 {
            n237 = property on="P1 King" class="Pict"() -> ("Position"=w315:T1)  [unwired: 2 in, 2 out]
          }
          frame #25 {
            n238 = property on="P1 King 2" class="Pict"() -> ("Position"=w316:T1)  [unwired: 2 in, 2 out]
          }
          frame #26 {
            n239 = property on="P1 King 3" class="Pict"() -> ("Position"=w317:T1)  [unwired: 2 in, 2 out]
          }
          frame #27 {
            n240 = property on="P1 King 4" class="Pict"() -> ("Position"=w318:T1)  [unwired: 2 in, 2 out]
          }
          frame #28 {
            n241 = property on="P1 King 5" class="Pict"() -> ("Position"=w319:T1)  [unwired: 2 in, 2 out]
          }
          frame #29 {
            n242 = property on="P1 King 6" class="Pict"() -> ("Position"=w320:T1)  [unwired: 2 in, 2 out]
          }
          frame #30 {
            n243 = property on="P1 King 7" class="Pict"() -> ("Position"=w321:T1)  [unwired: 2 in, 2 out]
          }
          frame #31 {
            n244 = property on="P1 King 8" class="Pict"() -> ("Position"=w322:T1)  [unwired: 2 in, 2 out]
          }
          frame #32 {
            n245 = property on="P1 King 9" class="Pict"() -> ("Position"=w323:T1)  [unwired: 2 in, 2 out]
          }
          frame #33 {
            n246 = property on="P1 King 10" class="Pict"() -> ("Position"=w324:T1)  [unwired: 2 in, 2 out]
          }
          frame #34 {
            n247 = property on="P1 King 11" class="Pict"() -> ("Position"=w325:T1)  [unwired: 2 in, 2 out]
          }
          frame #35 {
            n248 = property on="P1 King 12" class="Pict"() -> ("Position"=w326:T1)  [unwired: 2 in, 2 out]
          }
          frame #36 {
            n249 = property on="P2 King" class="Pict"() -> ("Position"=w327:T1)  [unwired: 2 in, 2 out]
          }
          frame #37 {
            n250 = property on="P2 King 2" class="Pict"() -> ("Position"=w328:T1)  [unwired: 2 in, 2 out]
          }
          frame #38 {
            n251 = property on="P2 King 3" class="Pict"() -> ("Position"=w329:T1)  [unwired: 2 in, 2 out]
          }
          frame #39 {
            n252 = property on="P2 King 4" class="Pict"() -> ("Position"=w330:T1)  [unwired: 2 in, 2 out]
          }
          frame #40 {
            n253 = property on="P2 King 5" class="Pict"() -> ("Position"=w331:T1)  [unwired: 2 in, 2 out]
          }
          frame #41 {
            n254 = property on="P2 King 6" class="Pict"() -> ("Position"=w332:T1)  [unwired: 2 in, 2 out]
          }
          frame #42 {
            n255 = property on="P2 King 7" class="Pict"() -> ("Position"=w333:T1)  [unwired: 2 in, 2 out]
          }
          frame #43 {
            n256 = property on="P2 King 8" class="Pict"() -> ("Position"=w334:T1)  [unwired: 2 in, 2 out]
          }
          frame #44 {
            n257 = property on="P2 King 9" class="Pict"() -> ("Position"=w335:T1)  [unwired: 2 in, 2 out]
          }
          frame #45 {
            n258 = property on="P2 King 10" class="Pict"() -> ("Position"=w336:T1)  [unwired: 2 in, 2 out]
          }
          frame #46 {
            n259 = property on="P2 King 11" class="Pict"() -> ("Position"=w337:T1)  [unwired: 2 in, 2 out]
          }
          frame #47 {
            n260 = property on="P2 King 12" class="Pict"() -> ("Position"=w338:T1)  [unwired: 2 in, 2 out]
          }
        }
        n261 = Build Array(w275, w274, w273, w272, w271, w270, w269, w268, w267, w266, w265, w264) -> (w263:T1[])
        n262 = Build Array (concatenate)(w263, w262, w261, w260, w259, w258, w257, w256, w255, w254, w253, w252, w251) -> (w250:T1[])
        n263 = Build Array (concatenate)(w250, w249, w248, w247, w246, w245, w244, w243, w242, w241, w240, w239, w238) -> (w237:T1[])
        n264 = Build Array (concatenate)(w237, w236, w235, w234, w233, w232, w231, w230, w229, w228, w227, w226, w225) -> (w224:T1[])
        n265 = for {
          tunnel: w224 -> [w346] mode=indexing
          tunnel: w288 -> [w345]
          n266 = Unbundle(w346) -> ("Left"=w340:i32, "Top"=w339:i32)
          n267 = Set File Position(refnum=w345, from (0:start)=enum16{"start", "end", "current"}."end") -> (refnum out=w342:refnum<file>)  [unwired: 2 in, 1 out]
          n268 = Format Into String(initial string=w342, " " ("input 1")) -> (resulting string=w341:refnum<file>)  [unwired: 2 in, 1 out]
          n269 = Format Into String(initial string=w341, w340, w339) -> ()  [unwired: 2 in, 2 out]
        }
      }
      event "Save and Quit": Value Change {
        n270 = event-data() -> ()  [unwired: 1 in, 6 out]
        n271 = flat-sequence {
          tunnel: [w348] -> w347
          frame #0 {
            n272 = global read "Game Info Global Variable.vi" "P1 King Text Green Color"() -> (w357:i32)
            n273 = global read "Game Info Global Variable.vi" "P2 King Text Green Color"() -> (w351:i32)
            n274 = global read "Game Info Global Variable.vi" "P1 King Text Blue Color"() -> (w356:i32)
            n275 = global read "Game Info Global Variable.vi" "P2 King Text Blue Color"() -> (w350:i32)
            n276 = global read "Game Info Global Variable.vi" "P1 King Text Red Color"() -> (w358:i32)
            n277 = global read "Game Info Global Variable.vi" "P2 King Text Red Color"() -> (w352:i32)
            n278 = global read "Game Info Global Variable.vi" "P1 Green Color"() -> (w360:i32)
            n279 = global read "Game Info Global Variable.vi" "P2 Green Color"() -> (w354:i32)
            n280 = local read "Player 1 Name"() -> (w363:string)
            n281 = local read "Player 2 Name"() -> (w362:string)
            n282 = global read "Game Info Global Variable.vi" "P1 Red Color"() -> (w361:i32)
            n283 = global read "Game Info Global Variable.vi" "P1 Blue Color"() -> (w359:i32)
            n284 = global read "Game Info Global Variable.vi" "P2 Blue Color"() -> (w353:i32)
            n285 = global read "Game Info Global Variable.vi" "P2 Red Color"() -> (w355:i32)
            n286 = Format Into String(w363, w362, w361, w360, w359, w358, w357, w356, w355, w354, w353, w352, w351, w350) -> (resulting string=w349:refnum<file>)  [unwired: 3 in, 1 out]
            n287 = stacked-sequence {
              tunnel: [w415 _ _ _ _ _ _ _ _ _ _ _ _ _ _ _ _ _ _ _ _ _ _ _ _ _ _ _ _ _ _ _ _ _ _ _ _ _ _ _ _ _ _ _ _ _ _ _] -> w364
              tunnel: [_ w416 _ _ _ _ _ _ _ _ _ _ _ _ _ _ _ _ _ _ _ _ _ _ _ _ _ _ _ _ _ _ _ _ _ _ _ _ _ _ _ _ _ _ _ _ _ _] -> w365
              tunnel: [_ _ w417 _ _ _ _ _ _ _ _ _ _ _ _ _ _ _ _ _ _ _ _ _ _ _ _ _ _ _ _ _ _ _ _ _ _ _ _ _ _ _ _ _ _ _ _ _] -> w366
              tunnel: [_ _ _ w418 _ _ _ _ _ _ _ _ _ _ _ _ _ _ _ _ _ _ _ _ _ _ _ _ _ _ _ _ _ _ _ _ _ _ _ _ _ _ _ _ _ _ _ _] -> w367
              tunnel: [_ _ _ _ w419 _ _ _ _ _ _ _ _ _ _ _ _ _ _ _ _ _ _ _ _ _ _ _ _ _ _ _ _ _ _ _ _ _ _ _ _ _ _ _ _ _ _ _] -> w368
              tunnel: [_ _ _ _ _ w420 _ _ _ _ _ _ _ _ _ _ _ _ _ _ _ _ _ _ _ _ _ _ _ _ _ _ _ _ _ _ _ _ _ _ _ _ _ _ _ _ _ _] -> w369
              tunnel: [_ _ _ _ _ _ w421 _ _ _ _ _ _ _ _ _ _ _ _ _ _ _ _ _ _ _ _ _ _ _ _ _ _ _ _ _ _ _ _ _ _ _ _ _ _ _ _ _] -> w370
              tunnel: [_ _ _ _ _ _ _ w422 _ _ _ _ _ _ _ _ _ _ _ _ _ _ _ _ _ _ _ _ _ _ _ _ _ _ _ _ _ _ _ _ _ _ _ _ _ _ _ _] -> w371
              tunnel: [_ _ _ _ _ _ _ _ w423 _ _ _ _ _ _ _ _ _ _ _ _ _ _ _ _ _ _ _ _ _ _ _ _ _ _ _ _ _ _ _ _ _ _ _ _ _ _ _] -> w372
              tunnel: [_ _ _ _ _ _ _ _ _ w424 _ _ _ _ _ _ _ _ _ _ _ _ _ _ _ _ _ _ _ _ _ _ _ _ _ _ _ _ _ _ _ _ _ _ _ _ _ _] -> w373
              tunnel: [_ _ _ _ _ _ _ _ _ _ w425 _ _ _ _ _ _ _ _ _ _ _ _ _ _ _ _ _ _ _ _ _ _ _ _ _ _ _ _ _ _ _ _ _ _ _ _ _] -> w374
              tunnel: [_ _ _ _ _ _ _ _ _ _ _ w426 _ _ _ _ _ _ _ _ _ _ _ _ _ _ _ _ _ _ _ _ _ _ _ _ _ _ _ _ _ _ _ _ _ _ _ _] -> w375
              tunnel: [_ _ _ _ _ _ _ _ _ _ _ _ w427 _ _ _ _ _ _ _ _ _ _ _ _ _ _ _ _ _ _ _ _ _ _ _ _ _ _ _ _ _ _ _ _ _ _ _] -> w377
              tunnel: [_ _ _ _ _ _ _ _ _ _ _ _ _ w428 _ _ _ _ _ _ _ _ _ _ _ _ _ _ _ _ _ _ _ _ _ _ _ _ _ _ _ _ _ _ _ _ _ _] -> w378
              tunnel: [_ _ _ _ _ _ _ _ _ _ _ _ _ _ w429 _ _ _ _ _ _ _ _ _ _ _ _ _ _ _ _ _ _ _ _ _ _ _ _ _ _ _ _ _ _ _ _ _] -> w379
              tunnel: [_ _ _ _ _ _ _ _ _ _ _ _ _ _ _ w430 _ _ _ _ _ _ _ _ _ _ _ _ _ _ _ _ _ _ _ _ _ _ _ _ _ _ _ _ _ _ _ _] -> w380
              tunnel: [_ _ _ _ _ _ _ _ _ _ _ _ _ _ _ _ w431 _ _ _ _ _ _ _ _ _ _ _ _ _ _ _ _ _ _ _ _ _ _ _ _ _ _ _ _ _ _ _] -> w381
              tunnel: [_ _ _ _ _ _ _ _ _ _ _ _ _ _ _ _ _ w432 _ _ _ _ _ _ _ _ _ _ _ _ _ _ _ _ _ _ _ _ _ _ _ _ _ _ _ _ _ _] -> w382
              tunnel: [_ _ _ _ _ _ _ _ _ _ _ _ _ _ _ _ _ _ w433 _ _ _ _ _ _ _ _ _ _ _ _ _ _ _ _ _ _ _ _ _ _ _ _ _ _ _ _ _] -> w383
              tunnel: [_ _ _ _ _ _ _ _ _ _ _ _ _ _ _ _ _ _ _ w434 _ _ _ _ _ _ _ _ _ _ _ _ _ _ _ _ _ _ _ _ _ _ _ _ _ _ _ _] -> w384
              tunnel: [_ _ _ _ _ _ _ _ _ _ _ _ _ _ _ _ _ _ _ _ w435 _ _ _ _ _ _ _ _ _ _ _ _ _ _ _ _ _ _ _ _ _ _ _ _ _ _ _] -> w385
              tunnel: [_ _ _ _ _ _ _ _ _ _ _ _ _ _ _ _ _ _ _ _ _ w436 _ _ _ _ _ _ _ _ _ _ _ _ _ _ _ _ _ _ _ _ _ _ _ _ _ _] -> w386
              tunnel: [_ _ _ _ _ _ _ _ _ _ _ _ _ _ _ _ _ _ _ _ _ _ w437 _ _ _ _ _ _ _ _ _ _ _ _ _ _ _ _ _ _ _ _ _ _ _ _ _] -> w388
              tunnel: [_ _ _ _ _ _ _ _ _ _ _ _ _ _ _ _ _ _ _ _ _ _ _ w438 _ _ _ _ _ _ _ _ _ _ _ _ _ _ _ _ _ _ _ _ _ _ _ _] -> w387
              tunnel: [_ _ _ _ _ _ _ _ _ _ _ _ _ _ _ _ _ _ _ _ _ _ _ _ w439 _ _ _ _ _ _ _ _ _ _ _ _ _ _ _ _ _ _ _ _ _ _ _] -> w391
              tunnel: [_ _ _ _ _ _ _ _ _ _ _ _ _ _ _ _ _ _ _ _ _ _ _ _ _ w440 _ _ _ _ _ _ _ _ _ _ _ _ _ _ _ _ _ _ _ _ _ _] -> w392
              tunnel: [_ _ _ _ _ _ _ _ _ _ _ _ _ _ _ _ _ _ _ _ _ _ _ _ _ _ w441 _ _ _ _ _ _ _ _ _ _ _ _ _ _ _ _ _ _ _ _ _] -> w393
              tunnel: [_ _ _ _ _ _ _ _ _ _ _ _ _ _ _ _ _ _ _ _ _ _ _ _ _ _ _ w442 _ _ _ _ _ _ _ _ _ _ _ _ _ _ _ _ _ _ _ _] -> w394
              tunnel: [_ _ _ _ _ _ _ _ _ _ _ _ _ _ _ _ _ _ _ _ _ _ _ _ _ _ _ _ w443 _ _ _ _ _ _ _ _ _ _ _ _ _ _ _ _ _ _ _] -> w395
              tunnel: [_ _ _ _ _ _ _ _ _ _ _ _ _ _ _ _ _ _ _ _ _ _ _ _ _ _ _ _ _ w444 _ _ _ _ _ _ _ _ _ _ _ _ _ _ _ _ _ _] -> w396
              tunnel: [_ _ _ _ _ _ _ _ _ _ _ _ _ _ _ _ _ _ _ _ _ _ _ _ _ _ _ _ _ _ w445 _ _ _ _ _ _ _ _ _ _ _ _ _ _ _ _ _] -> w397
              tunnel: [_ _ _ _ _ _ _ _ _ _ _ _ _ _ _ _ _ _ _ _ _ _ _ _ _ _ _ _ _ _ _ w446 _ _ _ _ _ _ _ _ _ _ _ _ _ _ _ _] -> w398
              tunnel: [_ _ _ _ _ _ _ _ _ _ _ _ _ _ _ _ _ _ _ _ _ _ _ _ _ _ _ _ _ _ _ _ w447 _ _ _ _ _ _ _ _ _ _ _ _ _ _ _] -> w399
              tunnel: [_ _ _ _ _ _ _ _ _ _ _ _ _ _ _ _ _ _ _ _ _ _ _ _ _ _ _ _ _ _ _ _ _ w448 _ _ _ _ _ _ _ _ _ _ _ _ _ _] -> w400
              tunnel: [_ _ _ _ _ _ _ _ _ _ _ _ _ _ _ _ _ _ _ _ _ _ _ _ _ _ _ _ _ _ _ _ _ _ w449 _ _ _ _ _ _ _ _ _ _ _ _ _] -> w401
              tunnel: [_ _ _ _ _ _ _ _ _ _ _ _ _ _ _ _ _ _ _ _ _ _ _ _ _ _ _ _ _ _ _ _ _ _ _ w450 _ _ _ _ _ _ _ _ _ _ _ _] -> w402
              tunnel: [_ _ _ _ _ _ _ _ _ _ _ _ _ _ _ _ _ _ _ _ _ _ _ _ _ _ _ _ _ _ _ _ _ _ _ _ w451 _ _ _ _ _ _ _ _ _ _ _] -> w403
              tunnel: [_ _ _ _ _ _ _ _ _ _ _ _ _ _ _ _ _ _ _ _ _ _ _ _ _ _ _ _ _ _ _ _ _ _ _ _ _ w452 _ _ _ _ _ _ _ _ _ _] -> w404
              tunnel: [_ _ _ _ _ _ _ _ _ _ _ _ _ _ _ _ _ _ _ _ _ _ _ _ _ _ _ _ _ _ _ _ _ _ _ _ _ _ w453 _ _ _ _ _ _ _ _ _] -> w405
              tunnel: [_ _ _ _ _ _ _ _ _ _ _ _ _ _ _ _ _ _ _ _ _ _ _ _ _ _ _ _ _ _ _ _ _ _ _ _ _ _ _ w454 _ _ _ _ _ _ _ _] -> w406
              tunnel: [_ _ _ _ _ _ _ _ _ _ _ _ _ _ _ _ _ _ _ _ _ _ _ _ _ _ _ _ _ _ _ _ _ _ _ _ _ _ _ _ w455 _ _ _ _ _ _ _] -> w407
              tunnel: [_ _ _ _ _ _ _ _ _ _ _ _ _ _ _ _ _ _ _ _ _ _ _ _ _ _ _ _ _ _ _ _ _ _ _ _ _ _ _ _ _ w456 _ _ _ _ _ _] -> w408
              tunnel: [_ _ _ _ _ _ _ _ _ _ _ _ _ _ _ _ _ _ _ _ _ _ _ _ _ _ _ _ _ _ _ _ _ _ _ _ _ _ _ _ _ _ w457 _ _ _ _ _] -> w409
              tunnel: [_ _ _ _ _ _ _ _ _ _ _ _ _ _ _ _ _ _ _ _ _ _ _ _ _ _ _ _ _ _ _ _ _ _ _ _ _ _ _ _ _ _ _ w458 _ _ _ _] -> w410
              tunnel: [_ _ _ _ _ _ _ _ _ _ _ _ _ _ _ _ _ _ _ _ _ _ _ _ _ _ _ _ _ _ _ _ _ _ _ _ _ _ _ _ _ _ _ _ w459 _ _ _] -> w411
              tunnel: [_ _ _ _ _ _ _ _ _ _ _ _ _ _ _ _ _ _ _ _ _ _ _ _ _ _ _ _ _ _ _ _ _ _ _ _ _ _ _ _ _ _ _ _ _ w460 _ _] -> w412
              tunnel: [_ _ _ _ _ _ _ _ _ _ _ _ _ _ _ _ _ _ _ _ _ _ _ _ _ _ _ _ _ _ _ _ _ _ _ _ _ _ _ _ _ _ _ _ _ _ w461 _] -> w413
              tunnel: [_ _ _ _ _ _ _ _ _ _ _ _ _ _ _ _ _ _ _ _ _ _ _ _ _ _ _ _ _ _ _ _ _ _ _ _ _ _ _ _ _ _ _ _ _ _ _ w462] -> w414
              frame #0 {
                n288 = property on="P1 Piece" class="Pict"() -> ("Position"=w415:T1)  [unwired: 2 in, 2 out]
              }
              frame #1 {
                n289 = property on="P1 Piece 2" class="Pict"() -> ("Position"=w416:T1)  [unwired: 2 in, 2 out]
              }
              frame #2 {
                n290 = property on="P1 Piece 3" class="Pict"() -> ("Position"=w417:T1)  [unwired: 2 in, 2 out]
              }
              frame #3 {
                n291 = property on="P1 Piece 4" class="Pict"() -> ("Position"=w418:T1)  [unwired: 2 in, 2 out]
              }
              frame #4 {
                n292 = property on="P1 Piece 5" class="Pict"() -> ("Position"=w419:T1)  [unwired: 2 in, 2 out]
              }
              frame #5 {
                n293 = property on="P1 Piece 6" class="Pict"() -> ("Position"=w420:T1)  [unwired: 2 in, 2 out]
              }
              frame #6 {
                n294 = property on="P1 Piece 7" class="Pict"() -> ("Position"=w421:T1)  [unwired: 2 in, 2 out]
              }
              frame #7 {
                n295 = property on="P1 Piece 8" class="Pict"() -> ("Position"=w422:T1)  [unwired: 2 in, 2 out]
              }
              frame #8 {
                n296 = property on="P1 Piece 9" class="Pict"() -> ("Position"=w423:T1)  [unwired: 2 in, 2 out]
              }
              frame #9 {
                n297 = property on="P1 Piece 10" class="Pict"() -> ("Position"=w424:T1)  [unwired: 2 in, 2 out]
              }
              frame #10 {
                n298 = property on="P1 Piece 11" class="Pict"() -> ("Position"=w425:T1)  [unwired: 2 in, 2 out]
              }
              frame #11 {
                n299 = property on="P1 Piece 12" class="Pict"() -> ("Position"=w426:T1)  [unwired: 2 in, 2 out]
              }
              frame #12 {
                n300 = property on="P2 Piece" class="Pict"() -> ("Position"=w427:T1)  [unwired: 2 in, 2 out]
              }
              frame #13 {
                n301 = property on="P2 Piece 2" class="Pict"() -> ("Position"=w428:T1)  [unwired: 2 in, 2 out]
              }
              frame #14 {
                n302 = property on="P2 Piece 3" class="Pict"() -> ("Position"=w429:T1)  [unwired: 2 in, 2 out]
              }
              frame #15 {
                n303 = property on="P2 Piece 4" class="Pict"() -> ("Position"=w430:T1)  [unwired: 2 in, 2 out]
              }
              frame #16 {
                n304 = property on="P2 Piece 5" class="Pict"() -> ("Position"=w431:T1)  [unwired: 2 in, 2 out]
              }
              frame #17 {
                n305 = property on="P2 Piece 6" class="Pict"() -> ("Position"=w432:T1)  [unwired: 2 in, 2 out]
              }
              frame #18 {
                n306 = property on="P2 Piece 7" class="Pict"() -> ("Position"=w433:T1)  [unwired: 2 in, 2 out]
              }
              frame #19 {
                n307 = property on="P2 Piece 8" class="Pict"() -> ("Position"=w434:T1)  [unwired: 2 in, 2 out]
              }
              frame #20 {
                n308 = property on="P2 Piece 9" class="Pict"() -> ("Position"=w435:T1)  [unwired: 2 in, 2 out]
              }
              frame #21 {
                n309 = property on="P2 Piece 10" class="Pict"() -> ("Position"=w436:T1)  [unwired: 2 in, 2 out]
              }
              frame #22 {
                n310 = property on="P2 Piece 11" class="Pict"() -> ("Position"=w437:T1)  [unwired: 2 in, 2 out]
              }
              frame #23 {
                n311 = property on="P2 Piece 12" class="Pict"() -> ("Position"=w438:T1)  [unwired: 2 in, 2 out]
              }
              frame #24 {
                n312 = property on="P1 King" class="Pict"() -> ("Position"=w439:T1)  [unwired: 2 in, 2 out]
              }
              frame #25 {
                n313 = property on="P1 King 2" class="Pict"() -> ("Position"=w440:T1)  [unwired: 2 in, 2 out]
              }
              frame #26 {
                n314 = property on="P1 King 3" class="Pict"() -> ("Position"=w441:T1)  [unwired: 2 in, 2 out]
              }
              frame #27 {
                n315 = property on="P1 King 4" class="Pict"() -> ("Position"=w442:T1)  [unwired: 2 in, 2 out]
              }
              frame #28 {
                n316 = property on="P1 King 5" class="Pict"() -> ("Position"=w443:T1)  [unwired: 2 in, 2 out]
              }
              frame #29 {
                n317 = property on="P1 King 6" class="Pict"() -> ("Position"=w444:T1)  [unwired: 2 in, 2 out]
              }
              frame #30 {
                n318 = property on="P1 King 7" class="Pict"() -> ("Position"=w445:T1)  [unwired: 2 in, 2 out]
              }
              frame #31 {
                n319 = property on="P1 King 8" class="Pict"() -> ("Position"=w446:T1)  [unwired: 2 in, 2 out]
              }
              frame #32 {
                n320 = property on="P1 King 9" class="Pict"() -> ("Position"=w447:T1)  [unwired: 2 in, 2 out]
              }
              frame #33 {
                n321 = property on="P1 King 10" class="Pict"() -> ("Position"=w448:T1)  [unwired: 2 in, 2 out]
              }
              frame #34 {
                n322 = property on="P1 King 11" class="Pict"() -> ("Position"=w449:T1)  [unwired: 2 in, 2 out]
              }
              frame #35 {
                n323 = property on="P1 King 12" class="Pict"() -> ("Position"=w450:T1)  [unwired: 2 in, 2 out]
              }
              frame #36 {
                n324 = property on="P2 King" class="Pict"() -> ("Position"=w451:T1)  [unwired: 2 in, 2 out]
              }
              frame #37 {
                n325 = property on="P2 King 2" class="Pict"() -> ("Position"=w452:T1)  [unwired: 2 in, 2 out]
              }
              frame #38 {
                n326 = property on="P2 King 3" class="Pict"() -> ("Position"=w453:T1)  [unwired: 2 in, 2 out]
              }
              frame #39 {
                n327 = property on="P2 King 4" class="Pict"() -> ("Position"=w454:T1)  [unwired: 2 in, 2 out]
              }
              frame #40 {
                n328 = property on="P2 King 5" class="Pict"() -> ("Position"=w455:T1)  [unwired: 2 in, 2 out]
              }
              frame #41 {
                n329 = property on="P2 King 6" class="Pict"() -> ("Position"=w456:T1)  [unwired: 2 in, 2 out]
              }
              frame #42 {
                n330 = property on="P2 King 7" class="Pict"() -> ("Position"=w457:T1)  [unwired: 2 in, 2 out]
              }
              frame #43 {
                n331 = property on="P2 King 8" class="Pict"() -> ("Position"=w458:T1)  [unwired: 2 in, 2 out]
              }
              frame #44 {
                n332 = property on="P2 King 9" class="Pict"() -> ("Position"=w459:T1)  [unwired: 2 in, 2 out]
              }
              frame #45 {
                n333 = property on="P2 King 10" class="Pict"() -> ("Position"=w460:T1)  [unwired: 2 in, 2 out]
              }
              frame #46 {
                n334 = property on="P2 King 11" class="Pict"() -> ("Position"=w461:T1)  [unwired: 2 in, 2 out]
              }
              frame #47 {
                n335 = property on="P2 King 12" class="Pict"() -> ("Position"=w462:T1)  [unwired: 2 in, 2 out]
              }
            }
            n336 = Build Array(w364, w365, w366, w367, w368, w369, w370, w371, w372, w373, w374, w375) -> (w376:T1[])
            n337 = Build Array (concatenate)(w376, w377, w378, w379, w380, w381, w382, w383, w384, w385, w386, w388, w387) -> (w389:T1[])
            n338 = Build Array (concatenate)(w389, w391, w392, w393, w394, w395, w396, w397, w398, w399, w400, w401, w402) -> (w390:T1[])
            n339 = Build Array (concatenate)(w390, w403, w404, w405, w406, w407, w408, w409, w410, w411, w412, w413, w414) -> (w348:T1[])
            n340 = for {
              tunnel: w348 -> [w470] mode=indexing
              tunnel: w349 -> [w469]
              n341 = Unbundle(w470) -> ("Left"=w464:i32, "Top"=w463:i32)
              n342 = Set File Position(refnum=w469, from (0:start)=enum16{"start", "end", "current"}."end") -> (refnum out=w466:refnum<file>)  [unwired: 2 in, 1 out]
              n343 = Format Into String(initial string=w466, " " ("input 1")) -> (resulting string=w465:refnum<file>)  [unwired: 2 in, 1 out]
              n344 = Format Into String(initial string=w465, w464, w463) -> ()  [unwired: 2 in, 2 out]
            }
          }
          frame #1 {
            n345 = vi-ref "Checkers Main Menu.vi"() -> (w474:refnum<vi>)
            n346 = vi-ref "Checkers Gymnopedie Music Player.vi"() -> (w471:refnum<vi>)
            n347 = invoke class="VI" method="Run VI"(reference=w474, "Wait until done"=FALSE ("Wait Until Done")) -> (reference out=w475:refnum<vi>, error out=w476:errorcluster)  [unwired: 3 in, 3 out]
            n348 = invoke class="VI" method="Run VI"(reference=w471, "Wait until done"=FALSE ("Wait Until Done")) -> ()  [unwired: 3 in, 5 out]
            n349 = invoke class="VI" method="FP.Open"(reference=w475, error in=w476, "Activate"=TRUE ("Activate?")) -> (error out=w477:errorcluster)  [unwired: 2 in, 4 out]
            n350 = vi-ref "Checkers Palladio Music Player.vi"() -> (w473:refnum<vi>)
            n351 = vi-ref "Checkers PvP.vi"() -> (w478:refnum<vi>)
            n352 = invoke class="VI" method="Abort VI"(reference=w478, error in=w477) -> ()  [unwired: 1 in, 3 out]
            n353 = invoke class="VI" method="Abort VI"(reference=w473) -> ()  [unwired: 2 in, 3 out]
          }
        }
      }
      event "Quit": Value Change {
        n354 = event-data() -> ()  [unwired: 1 in, 6 out]
        n355 = Two Button Dialog(message="Are you sure you want to quit without saving?", 1:"No" ("F button name (\"Cancel\")"), 2:"Yes" ("T button name (\"OK\")")) -> (T button?=w482:bool)
        n356 = case shown="False" w482 {
          frame False {
            # "Player changed mind to quit without saving. Do nothing."
          }
          frame True {
            n357 = vi-ref "Checkers Gymnopedie Music Player.vi"() -> (w486:refnum<vi>)
            n358 = vi-ref "Checkers Main Menu.vi"() -> (w495:refnum<vi>)
            n359 = invoke class="VI" method="Run VI"(reference=w495, "Wait until done"=FALSE ("Wait Until Done")) -> (reference out=w494:refnum<vi>, error out=w493:errorcluster)  [unwired: 3 in, 3 out]
            n360 = invoke class="VI" method="Run VI"(reference=w486, "Wait until done"=FALSE ("Wait Until Done")) -> ()  [unwired: 3 in, 5 out]
            n361 = invoke class="VI" method="FP.Open"(reference=w494, error in=w493, "Activate"=TRUE ("Activate?")) -> (error out=w492:errorcluster)  [unwired: 2 in, 4 out]
            n362 = vi-ref "Checkers Palladio Music Player.vi"() -> (w488:refnum<vi>)
            n363 = vi-ref "Checkers PvP.vi"() -> (w491:refnum<vi>)
            n364 = invoke class="VI" method="Abort VI"(reference=w491, error in=w492) -> ()  [unwired: 1 in, 3 out]
            n365 = invoke class="VI" method="Abort VI"(reference=w488) -> ()  [unwired: 2 in, 3 out]
          }
        }
      }
      event "P1 Piece 10", "P1 Piece 2", "P1 Piece 3", "P1 Piece 4", "P1 Piece 5", "P1 Piece 6", "P1 Piece 7", "P1 Piece 8", "P1 Piece 9", "P1 Piece 11", "P1 Piece 12": Mouse Down {
        n366 = event-data() -> ()  [unwired: 1 in, 8 out]
        n367 = local read "P1 Turn Light"() -> (w498:bool)
        n368 = case shown="True" w498 {
          tunnel: w497 -> [_ w502]
          tunnel: [_ w499] -> w496
          frame False {
            # "It's not player 1's turn yet. Do nothing."
          }
          frame True {
            # "At this point, I use an \nequation to turn the pixel\ncoordinates into the array coordinates\nof the piece that the user clicked."
            # "Left first"
            # "row[0], collumn[1]"
            n369 = global read "Board Layout Global Variable.vi" "Board Layout"() -> (w537:dbl[][])
            n370 = property on="P1 Piece 10" class="Pict"() -> ("Position"=w536:T1)  [unwired: 2 in, 2 out]
            n371 = Unbundle By Name(w536) -> ("Left"=w525:i32, "Top"=w523:i32)
            n372 = expression code="(x-469)/42"(w525) -> (w526:i32)
            n373 = expression code="(x-56)/42"(w523) -> (w524:i32)
            n374 = To Long Integer(number=w526) -> (32bit integer=w508:i32)
            n375 = To Long Integer(number=w524) -> (32bit integer=w509:i32)
            n376 = Build Array(w509, w508) -> (w535:i32[])
            n377 = call "MoveLogic.vi"("Coordinates"=w535, "Array"=w537) -> ("Moves"=w532:dbl[][])
            n378 = Index Array(array=w532, index (row)=0) -> (element=w510:dbl[])  [unwired: 1 in]
            n379 = Index Array(array=w532, index (row)=1) -> (element=w529:dbl[])  [unwired: 1 in]
            n380 = Index Array(array=w529, index=1) -> (element=w522:dbl)
            n381 = Index Array(array=w529, index=0) -> (element=w521:dbl)
            n382 = Index Array(array=w510, index=0) -> (element=w511:dbl)
            n383 = Index Array(array=w510, index=1) -> (element=w512:dbl)
            n384 = expression code="(x*42)+56"(w521) -> (w520:dbl)
            n385 = expression code="(x*42)+469"(w522) -> (w519:dbl)
            n386 = expression code="(x*42)+56"(w511) -> (w513:dbl)
            n387 = expression code="(x*42)+469"(w512) -> (w514:dbl)
            n388 = call <vilib>:"Three Button Dialog.vi"("Right Button Text (\"Cancel\")"="NOPE. GO BACK." ("Left Button Text (\"Yes\")"), "Center Button Text (\"No\")"="RIGHT" ("Left Button Text (\"Yes\")"), "Left Button Text (\"Yes\")"="LEFT" ("Left Button Text (\"Yes\")"), "message"="HOW YOU WANT MOVE?") -> ("Which Button?"=w506:T2)  [unwired: 7 in]
            n389 = To Long Integer(number=w519) -> (32bit integer=w518:i32)
            n390 = To Long Integer(number=w520) -> (32bit integer=w517:i32)
            n391 = case shown="\"Left Button\", Default" w506 {
              frame "Left Button", Default {
                n392 = property on="P1 Top Left Marker" class="Pict"() -> ("Position"=w544:T1)  [unwired: 2 in, 2 out]
                n393 = local read "P2 Turn Light"() -> (w541:bool)
                n394 = local read "P1 Turn Light"() -> (w539:bool)
                n395 = Not(x=w541) -> (.not. x?=w542:bool)
                n396 = Not(x=w539) -> (.not. x?=w540:bool)
                n397 = property on="P1 Top Right Marker" class="Pict"("Position"=T1 {"Left"=666, "Top"=666}) -> ()  [unwired: 2 in, 2 out]
                n398 = property on="P1 Piece 10" class="Pict"("Position"=w544) -> (error out=w543:errorcluster)  [unwired: 2 in, 1 out]
                n399 = property on="P1 Top Left Marker" class="Pict"(error in=w543, "Position"=T1 {"Left"=666, "Top"=666}) -> ()  [unwired: 1 in, 2 out]
                n400 = local write "P2 Turn Light"(w542) -> ()
                n401 = local write "P1 Turn Light"(w540) -> ()
              }
              frame "Right Button" {
                n402 = property on="P1 Top Left Marker" class="Pict"("Position"=T1 {"Left"=666, "Top"=666}) -> ()  [unwired: 2 in, 2 out]
                n403 = property on="P1 Top Right Marker" class="Pict"("Position"=T1 {"Left"=666, "Top"=666}) -> ()  [unwired: 2 in, 2 out]
              }
              frame "Center Button" {
                n404 = property on="P1 Top Right Marker" class="Pict"() -> ("Position"=w554:T1)  [unwired: 2 in, 2 out]
                n405 = local read "P2 Turn Light"() -> (w551:bool)
                n406 = local read "P1 Turn Light"() -> (w549:bool)
                n407 = Not(x=w551) -> (.not. x?=w552:bool)
                n408 = Not(x=w549) -> (.not. x?=w550:bool)
                n409 = property on="P1 Top Left Marker" class="Pict"("Position"=T1 {"Left"=666, "Top"=666}) -> ()  [unwired: 2 in, 2 out]
                n410 = property on="P1 Piece 10" class="Pict"("Position"=w554) -> (error out=w553:errorcluster)  [unwired: 2 in, 1 out]
                n411 = property on="P1 Top Right Marker" class="Pict"(error in=w553, "Position"=T1 {"Left"=666, "Top"=666}) -> ()  [unwired: 1 in, 2 out]
                n412 = local write "P2 Turn Light"(w552) -> ()
                n413 = local write "P1 Turn Light"(w550) -> ()
              }
            }
            n414 = To Long Integer(number=w514) -> (32bit integer=w515:i32)
            n415 = To Long Integer(number=w513) -> (32bit integer=w516:i32)
            n416 = Bundle(w518, w517) -> (w501:cluster{i32, i32})  [unwired: 1 in]
            n417 = Bundle(w515, w516) -> (w500:cluster{i32, i32})  [unwired: 1 in]
            n418 = property on="P1 Top Right Marker" class="Pict"("Position"=w501) -> ()  [unwired: 2 in, 2 out]
            n419 = property on="P1 Top Left Marker" class="Pict"("Position"=w500) -> ()  [unwired: 2 in, 2 out]
            n420 = for {
              tunnel: w502 -> [w538] mode=indexing
              tunnel: w501 -> [_]
              tunnel: w500 -> [_]
              tunnel: [w538] -> w499 mode=indexing
            }
          }
        }
      }
      event "P2 Piece 2": Mouse Down {
        n421 = event-data() -> ()  [unwired: 1 in, 8 out]
        n422 = local read "P1 Turn Light"() -> (w558:bool)
        n423 = case shown="True" w558 {
          frame False {
            # "It's not player 1's turn yet. Do nothing."
          }
          frame True {
            n424 = call "Checkers P1 Turn Drawer.vi"() -> ()  [unwired: 11 in, 1 out]
            n425 = stacked-sequence {
              tunnel: [w610 _ _ _ _ _ _ _ _ _ _ _ _ _ _ _ _ _ _ _ _ _ _ _ _ _ _ _ _ _ _ _ _ _ _ _ _ _ _ _ _ _ _ _ _ _ _ _] -> w609
              tunnel: [_ w611 _ _ _ _ _ _ _ _ _ _ _ _ _ _ _ _ _ _ _ _ _ _ _ _ _ _ _ _ _ _ _ _ _ _ _ _ _ _ _ _ _ _ _ _ _ _] -> w608
              tunnel: [_ _ w612 _ _ _ _ _ _ _ _ _ _ _ _ _ _ _ _ _ _ _ _ _ _ _ _ _ _ _ _ _ _ _ _ _ _ _ _ _ _ _ _ _ _ _ _ _] -> w607
              tunnel: [_ _ _ w613 _ _ _ _ _ _ _ _ _ _ _ _ _ _ _ _ _ _ _ _ _ _ _ _ _ _ _ _ _ _ _ _ _ _ _ _ _ _ _ _ _ _ _ _] -> w606
              tunnel: [_ _ _ _ w614 _ _ _ _ _ _ _ _ _ _ _ _ _ _ _ _ _ _ _ _ _ _ _ _ _ _ _ _ _ _ _ _ _ _ _ _ _ _ _ _ _ _ _] -> w605
              tunnel: [_ _ _ _ _ w615 _ _ _ _ _ _ _ _ _ _ _ _ _ _ _ _ _ _ _ _ _ _ _ _ _ _ _ _ _ _ _ _ _ _ _ _ _ _ _ _ _ _] -> w604
              tunnel: [_ _ _ _ _ _ w616 _ _ _ _ _ _ _ _ _ _ _ _ _ _ _ _ _ _ _ _ _ _ _ _ _ _ _ _ _ _ _ _ _ _ _ _ _ _ _ _ _] -> w603
              tunnel: [_ _ _ _ _ _ _ w617 _ _ _ _ _ _ _ _ _ _ _ _ _ _ _ _ _ _ _ _ _ _ _ _ _ _ _ _ _ _ _ _ _ _ _ _ _ _ _ _] -> w602
              tunnel: [_ _ _ _ _ _ _ _ w618 _ _ _ _ _ _ _ _ _ _ _ _ _ _ _ _ _ _ _ _ _ _ _ _ _ _ _ _ _ _ _ _ _ _ _ _ _ _ _] -> w601
              tunnel: [_ _ _ _ _ _ _ _ _ w619 _ _ _ _ _ _ _ _ _ _ _ _ _ _ _ _ _ _ _ _ _ _ _ _ _ _ _ _ _ _ _ _ _ _ _ _ _ _] -> w600
              tunnel: [_ _ _ _ _ _ _ _ _ _ w620 _ _ _ _ _ _ _ _ _ _ _ _ _ _ _ _ _ _ _ _ _ _ _ _ _ _ _ _ _ _ _ _ _ _ _ _ _] -> w599
              tunnel: [_ _ _ _ _ _ _ _ _ _ _ w621 _ _ _ _ _ _ _ _ _ _ _ _ _ _ _ _ _ _ _ _ _ _ _ _ _ _ _ _ _ _ _ _ _ _ _ _] -> w598
              tunnel: [_ _ _ _ _ _ _ _ _ _ _ _ w622 _ _ _ _ _ _ _ _ _ _ _ _ _ _ _ _ _ _ _ _ _ _ _ _ _ _ _ _ _ _ _ _ _ _ _] -> w596
              tunnel: [_ _ _ _ _ _ _ _ _ _ _ _ _ w623 _ _ _ _ _ _ _ _ _ _ _ _ _ _ _ _ _ _ _ _ _ _ _ _ _ _ _ _ _ _ _ _ _ _] -> w595
              tunnel: [_ _ _ _ _ _ _ _ _ _ _ _ _ _ w624 _ _ _ _ _ _ _ _ _ _ _ _ _ _ _ _ _ _ _ _ _ _ _ _ _ _ _ _ _ _ _ _ _] -> w594
              tunnel: [_ _ _ _ _ _ _ _ _ _ _ _ _ _ _ w625 _ _ _ _ _ _ _ _ _ _ _ _ _ _ _ _ _ _ _ _ _ _ _ _ _ _ _ _ _ _ _ _] -> w593
              tunnel: [_ _ _ _ _ _ _ _ _ _ _ _ _ _ _ _ w626 _ _ _ _ _ _ _ _ _ _ _ _ _ _ _ _ _ _ _ _ _ _ _ _ _ _ _ _ _ _ _] -> w592
              tunnel: [_ _ _ _ _ _ _ _ _ _ _ _ _ _ _ _ _ w627 _ _ _ _ _ _ _ _ _ _ _ _ _ _ _ _ _ _ _ _ _ _ _ _ _ _ _ _ _ _] -> w591
              tunnel: [_ _ _ _ _ _ _ _ _ _ _ _ _ _ _ _ _ _ w628 _ _ _ _ _ _ _ _ _ _ _ _ _ _ _ _ _ _ _ _ _ _ _ _ _ _ _ _ _] -> w590
              tunnel: [_ _ _ _ _ _ _ _ _ _ _ _ _ _ _ _ _ _ _ w629 _ _ _ _ _ _ _ _ _ _ _ _ _ _ _ _ _ _ _ _ _ _ _ _ _ _ _ _] -> w589
              tunnel: [_ _ _ _ _ _ _ _ _ _ _ _ _ _ _ _ _ _ _ _ w630 _ _ _ _ _ _ _ _ _ _ _ _ _ _ _ _ _ _ _ _ _ _ _ _ _ _ _] -> w588
              tunnel: [_ _ _ _ _ _ _ _ _ _ _ _ _ _ _ _ _ _ _ _ _ w631 _ _ _ _ _ _ _ _ _ _ _ _ _ _ _ _ _ _ _ _ _ _ _ _ _ _] -> w587
              tunnel: [_ _ _ _ _ _ _ _ _ _ _ _ _ _ _ _ _ _ _ _ _ _ w632 _ _ _ _ _ _ _ _ _ _ _ _ _ _ _ _ _ _ _ _ _ _ _ _ _] -> w585
              tunnel: [_ _ _ _ _ _ _ _ _ _ _ _ _ _ _ _ _ _ _ _ _ _ _ w633 _ _ _ _ _ _ _ _ _ _ _ _ _ _ _ _ _ _ _ _ _ _ _ _] -> w586
              tunnel: [_ _ _ _ _ _ _ _ _ _ _ _ _ _ _ _ _ _ _ _ _ _ _ _ w634 _ _ _ _ _ _ _ _ _ _ _ _ _ _ _ _ _ _ _ _ _ _ _] -> w582
              tunnel: [_ _ _ _ _ _ _ _ _ _ _ _ _ _ _ _ _ _ _ _ _ _ _ _ _ w635 _ _ _ _ _ _ _ _ _ _ _ _ _ _ _ _ _ _ _ _ _ _] -> w581
              tunnel: [_ _ _ _ _ _ _ _ _ _ _ _ _ _ _ _ _ _ _ _ _ _ _ _ _ _ w636 _ _ _ _ _ _ _ _ _ _ _ _ _ _ _ _ _ _ _ _ _] -> w580
              tunnel: [_ _ _ _ _ _ _ _ _ _ _ _ _ _ _ _ _ _ _ _ _ _ _ _ _ _ _ w637 _ _ _ _ _ _ _ _ _ _ _ _ _ _ _ _ _ _ _ _] -> w579
              tunnel: [_ _ _ _ _ _ _ _ _ _ _ _ _ _ _ _ _ _ _ _ _ _ _ _ _ _ _ _ w638 _ _ _ _ _ _ _ _ _ _ _ _ _ _ _ _ _ _ _] -> w578
              tunnel: [_ _ _ _ _ _ _ _ _ _ _ _ _ _ _ _ _ _ _ _ _ _ _ _ _ _ _ _ _ w639 _ _ _ _ _ _ _ _ _ _ _ _ _ _ _ _ _ _] -> w577
              tunnel: [_ _ _ _ _ _ _ _ _ _ _ _ _ _ _ _ _ _ _ _ _ _ _ _ _ _ _ _ _ _ w640 _ _ _ _ _ _ _ _ _ _ _ _ _ _ _ _ _] -> w576
              tunnel: [_ _ _ _ _ _ _ _ _ _ _ _ _ _ _ _ _ _ _ _ _ _ _ _ _ _ _ _ _ _ _ w641 _ _ _ _ _ _ _ _ _ _ _ _ _ _ _ _] -> w575
              tunnel: [_ _ _ _ _ _ _ _ _ _ _ _ _ _ _ _ _ _ _ _ _ _ _ _ _ _ _ _ _ _ _ _ w642 _ _ _ _ _ _ _ _ _ _ _ _ _ _ _] -> w574
              tunnel: [_ _ _ _ _ _ _ _ _ _ _ _ _ _ _ _ _ _ _ _ _ _ _ _ _ _ _ _ _ _ _ _ _ w643 _ _ _ _ _ _ _ _ _ _ _ _ _ _] -> w573
              tunnel: [_ _ _ _ _ _ _ _ _ _ _ _ _ _ _ _ _ _ _ _ _ _ _ _ _ _ _ _ _ _ _ _ _ _ w644 _ _ _ _ _ _ _ _ _ _ _ _ _] -> w572
              tunnel: [_ _ _ _ _ _ _ _ _ _ _ _ _ _ _ _ _ _ _ _ _ _ _ _ _ _ _ _ _ _ _ _ _ _ _ w645 _ _ _ _ _ _ _ _ _ _ _ _] -> w571
              tunnel: [_ _ _ _ _ _ _ _ _ _ _ _ _ _ _ _ _ _ _ _ _ _ _ _ _ _ _ _ _ _ _ _ _ _ _ _ w646 _ _ _ _ _ _ _ _ _ _ _] -> w570
              tunnel: [_ _ _ _ _ _ _ _ _ _ _ _ _ _ _ _ _ _ _ _ _ _ _ _ _ _ _ _ _ _ _ _ _ _ _ _ _ w647 _ _ _ _ _ _ _ _ _ _] -> w569
              tunnel: [_ _ _ _ _ _ _ _ _ _ _ _ _ _ _ _ _ _ _ _ _ _ _ _ _ _ _ _ _ _ _ _ _ _ _ _ _ _ w648 _ _ _ _ _ _ _ _ _] -> w568
              tunnel: [_ _ _ _ _ _ _ _ _ _ _ _ _ _ _ _ _ _ _ _ _ _ _ _ _ _ _ _ _ _ _ _ _ _ _ _ _ _ _ w649 _ _ _ _ _ _ _ _] -> w567
              tunnel: [_ _ _ _ _ _ _ _ _ _ _ _ _ _ _ _ _ _ _ _ _ _ _ _ _ _ _ _ _ _ _ _ _ _ _ _ _ _ _ _ w650 _ _ _ _ _ _ _] -> w566
              tunnel: [_ _ _ _ _ _ _ _ _ _ _ _ _ _ _ _ _ _ _ _ _ _ _ _ _ _ _ _ _ _ _ _ _ _ _ _ _ _ _ _ _ w651 _ _ _ _ _ _] -> w565
              tunnel: [_ _ _ _ _ _ _ _ _ _ _ _ _ _ _ _ _ _ _ _ _ _ _ _ _ _ _ _ _ _ _ _ _ _ _ _ _ _ _ _ _ _ w652 _ _ _ _ _] -> w564
              tunnel: [_ _ _ _ _ _ _ _ _ _ _ _ _ _ _ _ _ _ _ _ _ _ _ _ _ _ _ _ _ _ _ _ _ _ _ _ _ _ _ _ _ _ _ w653 _ _ _ _] -> w563
              tunnel: [_ _ _ _ _ _ _ _ _ _ _ _ _ _ _ _ _ _ _ _ _ _ _ _ _ _ _ _ _ _ _ _ _ _ _ _ _ _ _ _ _ _ _ _ w654 _ _ _] -> w562
              tunnel: [_ _ _ _ _ _ _ _ _ _ _ _ _ _ _ _ _ _ _ _ _ _ _ _ _ _ _ _ _ _ _ _ _ _ _ _ _ _ _ _ _ _ _ _ _ w655 _ _] -> w561
              tunnel: [_ _ _ _ _ _ _ _ _ _ _ _ _ _ _ _ _ _ _ _ _ _ _ _ _ _ _ _ _ _ _ _ _ _ _ _ _ _ _ _ _ _ _ _ _ _ w656 _] -> w560
              tunnel: [_ _ _ _ _ _ _ _ _ _ _ _ _ _ _ _ _ _ _ _ _ _ _ _ _ _ _ _ _ _ _ _ _ _ _ _ _ _ _ _ _ _ _ _ _ _ _ w657] -> w559
              frame #0 {
                n426 = property on="P1 Piece" class="Pict"() -> ("Position"=w610:T1)  [unwired: 2 in, 2 out]
              }
              frame #1 {
                n427 = property on="P1 Piece 2" class="Pict"() -> ("Position"=w611:T1)  [unwired: 2 in, 2 out]
              }
              frame #2 {
                n428 = property on="P1 Piece 3" class="Pict"() -> ("Position"=w612:T1)  [unwired: 2 in, 2 out]
              }
              frame #3 {
                n429 = property on="P1 Piece 4" class="Pict"() -> ("Position"=w613:T1)  [unwired: 2 in, 2 out]
              }
              frame #4 {
                n430 = property on="P1 Piece 5" class="Pict"() -> ("Position"=w614:T1)  [unwired: 2 in, 2 out]
              }
              frame #5 {
                n431 = property on="P1 Piece 6" class="Pict"() -> ("Position"=w615:T1)  [unwired: 2 in, 2 out]
              }
              frame #6 {
                n432 = property on="P1 Piece 7" class="Pict"() -> ("Position"=w616:T1)  [unwired: 2 in, 2 out]
              }
              frame #7 {
                n433 = property on="P1 Piece 8" class="Pict"() -> ("Position"=w617:T1)  [unwired: 2 in, 2 out]
              }
              frame #8 {
                n434 = property on="P1 Piece 9" class="Pict"() -> ("Position"=w618:T1)  [unwired: 2 in, 2 out]
              }
              frame #9 {
                n435 = property on="P1 Piece 10" class="Pict"() -> ("Position"=w619:T1)  [unwired: 2 in, 2 out]
              }
              frame #10 {
                n436 = property on="P1 Piece 11" class="Pict"() -> ("Position"=w620:T1)  [unwired: 2 in, 2 out]
              }
              frame #11 {
                n437 = property on="P1 Piece 12" class="Pict"() -> ("Position"=w621:T1)  [unwired: 2 in, 2 out]
              }
              frame #12 {
                n438 = property on="P2 Piece" class="Pict"() -> ("Position"=w622:T1)  [unwired: 2 in, 2 out]
              }
              frame #13 {
                n439 = property on="P2 Piece 2" class="Pict"() -> ("Position"=w623:T1)  [unwired: 2 in, 2 out]
              }
              frame #14 {
                n440 = property on="P2 Piece 3" class="Pict"() -> ("Position"=w624:T1)  [unwired: 2 in, 2 out]
              }
              frame #15 {
                n441 = property on="P2 Piece 4" class="Pict"() -> ("Position"=w625:T1)  [unwired: 2 in, 2 out]
              }
              frame #16 {
                n442 = property on="P2 Piece 5" class="Pict"() -> ("Position"=w626:T1)  [unwired: 2 in, 2 out]
              }
              frame #17 {
                n443 = property on="P2 Piece 6" class="Pict"() -> ("Position"=w627:T1)  [unwired: 2 in, 2 out]
              }
              frame #18 {
                n444 = property on="P2 Piece 7" class="Pict"() -> ("Position"=w628:T1)  [unwired: 2 in, 2 out]
              }
              frame #19 {
                n445 = property on="P2 Piece 8" class="Pict"() -> ("Position"=w629:T1)  [unwired: 2 in, 2 out]
              }
              frame #20 {
                n446 = property on="P2 Piece 9" class="Pict"() -> ("Position"=w630:T1)  [unwired: 2 in, 2 out]
              }
              frame #21 {
                n447 = property on="P2 Piece 10" class="Pict"() -> ("Position"=w631:T1)  [unwired: 2 in, 2 out]
              }
              frame #22 {
                n448 = property on="P2 Piece 11" class="Pict"() -> ("Position"=w632:T1)  [unwired: 2 in, 2 out]
              }
              frame #23 {
                n449 = property on="P2 Piece 12" class="Pict"() -> ("Position"=w633:T1)  [unwired: 2 in, 2 out]
              }
              frame #24 {
                n450 = property on="P1 King" class="Pict"() -> ("Position"=w634:T1)  [unwired: 2 in, 2 out]
              }
              frame #25 {
                n451 = property on="P1 King 2" class="Pict"() -> ("Position"=w635:T1)  [unwired: 2 in, 2 out]
              }
              frame #26 {
                n452 = property on="P1 King 3" class="Pict"() -> ("Position"=w636:T1)  [unwired: 2 in, 2 out]
              }
              frame #27 {
                n453 = property on="P1 King 4" class="Pict"() -> ("Position"=w637:T1)  [unwired: 2 in, 2 out]
              }
              frame #28 {
                n454 = property on="P1 King 5" class="Pict"() -> ("Position"=w638:T1)  [unwired: 2 in, 2 out]
              }
              frame #29 {
                n455 = property on="P1 King 6" class="Pict"() -> ("Position"=w639:T1)  [unwired: 2 in, 2 out]
              }
              frame #30 {
                n456 = property on="P1 King 7" class="Pict"() -> ("Position"=w640:T1)  [unwired: 2 in, 2 out]
              }
              frame #31 {
                n457 = property on="P1 King 8" class="Pict"() -> ("Position"=w641:T1)  [unwired: 2 in, 2 out]
              }
              frame #32 {
                n458 = property on="P1 King 9" class="Pict"() -> ("Position"=w642:T1)  [unwired: 2 in, 2 out]
              }
              frame #33 {
                n459 = property on="P1 King 10" class="Pict"() -> ("Position"=w643:T1)  [unwired: 2 in, 2 out]
              }
              frame #34 {
                n460 = property on="P1 King 11" class="Pict"() -> ("Position"=w644:T1)  [unwired: 2 in, 2 out]
              }
              frame #35 {
                n461 = property on="P1 King 12" class="Pict"() -> ("Position"=w645:T1)  [unwired: 2 in, 2 out]
              }
              frame #36 {
                n462 = property on="P2 King" class="Pict"() -> ("Position"=w646:T1)  [unwired: 2 in, 2 out]
              }
              frame #37 {
                n463 = property on="P2 King 2" class="Pict"() -> ("Position"=w647:T1)  [unwired: 2 in, 2 out]
              }
              frame #38 {
                n464 = property on="P2 King 3" class="Pict"() -> ("Position"=w648:T1)  [unwired: 2 in, 2 out]
              }
              frame #39 {
                n465 = property on="P2 King 4" class="Pict"() -> ("Position"=w649:T1)  [unwired: 2 in, 2 out]
              }
              frame #40 {
                n466 = property on="P2 King 5" class="Pict"() -> ("Position"=w650:T1)  [unwired: 2 in, 2 out]
              }
              frame #41 {
                n467 = property on="P2 King 6" class="Pict"() -> ("Position"=w651:T1)  [unwired: 2 in, 2 out]
              }
              frame #42 {
                n468 = property on="P2 King 7" class="Pict"() -> ("Position"=w652:T1)  [unwired: 2 in, 2 out]
              }
              frame #43 {
                n469 = property on="P2 King 8" class="Pict"() -> ("Position"=w653:T1)  [unwired: 2 in, 2 out]
              }
              frame #44 {
                n470 = property on="P2 King 9" class="Pict"() -> ("Position"=w654:T1)  [unwired: 2 in, 2 out]
              }
              frame #45 {
                n471 = property on="P2 King 10" class="Pict"() -> ("Position"=w655:T1)  [unwired: 2 in, 2 out]
              }
              frame #46 {
                n472 = property on="P2 King 11" class="Pict"() -> ("Position"=w656:T1)  [unwired: 2 in, 2 out]
              }
              frame #47 {
                n473 = property on="P2 King 12" class="Pict"() -> ("Position"=w657:T1)  [unwired: 2 in, 2 out]
              }
            }
            n474 = Build Array(w609, w608, w607, w606, w605, w604, w603, w602, w601, w600, w599, w598) -> (w597:T1[])
            n475 = Build Array (concatenate)(w597, w596, w595, w594, w593, w592, w591, w590, w589, w588, w587, w585, w586) -> (w584:T1[])
            n476 = Build Array (concatenate)(w584, w582, w581, w580, w579, w578, w577, w576, w575, w574, w573, w572, w571) -> (w583:T1[])
            n477 = Build Array (concatenate)(w583, w570, w569, w568, w567, w566, w565, w564, w563, w562, w561, w560, w559) -> ()  [unwired: 1 out]
          }
        }
      }
      event "P1 King": Mouse Down {
        n478 = event-data() -> ()  [unwired: 1 in, 8 out]
        n479 = local read "P1 Turn Light"() -> (w659:bool)
        n480 = case shown="True" w659 {
          frame False {
            # "It's not player 1's turn yet. Do nothing."
          }
          frame True {
            n481 = call "Checkers P1 Turn Drawer.vi"() -> ()  [unwired: 11 in, 1 out]
            n482 = stacked-sequence {
              tunnel: [w711 _ _ _ _ _ _ _ _ _ _ _ _ _ _ _ _ _ _ _ _ _ _ _ _ _ _ _ _ _ _ _ _ _ _ _ _ _ _ _ _ _ _ _ _ _ _ _] -> w710
              tunnel: [_ w712 _ _ _ _ _ _ _ _ _ _ _ _ _ _ _ _ _ _ _ _ _ _ _ _ _ _ _ _ _ _ _ _ _ _ _ _ _ _ _ _ _ _ _ _ _ _] -> w709
              tunnel: [_ _ w713 _ _ _ _ _ _ _ _ _ _ _ _ _ _ _ _ _ _ _ _ _ _ _ _ _ _ _ _ _ _ _ _ _ _ _ _ _ _ _ _ _ _ _ _ _] -> w708
              tunnel: [_ _ _ w714 _ _ _ _ _ _ _ _ _ _ _ _ _ _ _ _ _ _ _ _ _ _ _ _ _ _ _ _ _ _ _ _ _ _ _ _ _ _ _ _ _ _ _ _] -> w707
              tunnel: [_ _ _ _ w715 _ _ _ _ _ _ _ _ _ _ _ _ _ _ _ _ _ _ _ _ _ _ _ _ _ _ _ _ _ _ _ _ _ _ _ _ _ _ _ _ _ _ _] -> w706
              tunnel: [_ _ _ _ _ w716 _ _ _ _ _ _ _ _ _ _ _ _ _ _ _ _ _ _ _ _ _ _ _ _ _ _ _ _ _ _ _ _ _ _ _ _ _ _ _ _ _ _] -> w705
              tunnel: [_ _ _ _ _ _ w717 _ _ _ _ _ _ _ _ _ _ _ _ _ _ _ _ _ _ _ _ _ _ _ _ _ _ _ _ _ _ _ _ _ _ _ _ _ _ _ _ _] -> w704
              tunnel: [_ _ _ _ _ _ _ w718 _ _ _ _ _ _ _ _ _ _ _ _ _ _ _ _ _ _ _ _ _ _ _ _ _ _ _ _ _ _ _ _ _ _ _ _ _ _ _ _] -> w703
              tunnel: [_ _ _ _ _ _ _ _ w719 _ _ _ _ _ _ _ _ _ _ _ _ _ _ _ _ _ _ _ _ _ _ _ _ _ _ _ _ _ _ _ _ _ _ _ _ _ _ _] -> w702
              tunnel: [_ _ _ _ _ _ _ _ _ w720 _ _ _ _ _ _ _ _ _ _ _ _ _ _ _ _ _ _ _ _ _ _ _ _ _ _ _ _ _ _ _ _ _ _ _ _ _ _] -> w701
              tunnel: [_ _ _ _ _ _ _ _ _ _ w721 _ _ _ _ _ _ _ _ _ _ _ _ _ _ _ _ _ _ _ _ _ _ _ _ _ _ _ _ _ _ _ _ _ _ _ _ _] -> w700
              tunnel: [_ _ _ _ _ _ _ _ _ _ _ w722 _ _ _ _ _ _ _ _ _ _ _ _ _ _ _ _ _ _ _ _ _ _ _ _ _ _ _ _ _ _ _ _ _ _ _ _] -> w699
              tunnel: [_ _ _ _ _ _ _ _ _ _ _ _ w723 _ _ _ _ _ _ _ _ _ _ _ _ _ _ _ _ _ _ _ _ _ _ _ _ _ _ _ _ _ _ _ _ _ _ _] -> w697
              tunnel: [_ _ _ _ _ _ _ _ _ _ _ _ _ w724 _ _ _ _ _ _ _ _ _ _ _ _ _ _ _ _ _ _ _ _ _ _ _ _ _ _ _ _ _ _ _ _ _ _] -> w696
              tunnel: [_ _ _ _ _ _ _ _ _ _ _ _ _ _ w725 _ _ _ _ _ _ _ _ _ _ _ _ _ _ _ _ _ _ _ _ _ _ _ _ _ _ _ _ _ _ _ _ _] -> w695
              tunnel: [_ _ _ _ _ _ _ _ _ _ _ _ _ _ _ w726 _ _ _ _ _ _ _ _ _ _ _ _ _ _ _ _ _ _ _ _ _ _ _ _ _ _ _ _ _ _ _ _] -> w694
              tunnel: [_ _ _ _ _ _ _ _ _ _ _ _ _ _ _ _ w727 _ _ _ _ _ _ _ _ _ _ _ _ _ _ _ _ _ _ _ _ _ _ _ _ _ _ _ _ _ _ _] -> w693
              tunnel: [_ _ _ _ _ _ _ _ _ _ _ _ _ _ _ _ _ w728 _ _ _ _ _ _ _ _ _ _ _ _ _ _ _ _ _ _ _ _ _ _ _ _ _ _ _ _ _ _] -> w692
              tunnel: [_ _ _ _ _ _ _ _ _ _ _ _ _ _ _ _ _ _ w729 _ _ _ _ _ _ _ _ _ _ _ _ _ _ _ _ _ _ _ _ _ _ _ _ _ _ _ _ _] -> w691
              tunnel: [_ _ _ _ _ _ _ _ _ _ _ _ _ _ _ _ _ _ _ w730 _ _ _ _ _ _ _ _ _ _ _ _ _ _ _ _ _ _ _ _ _ _ _ _ _ _ _ _] -> w690
              tunnel: [_ _ _ _ _ _ _ _ _ _ _ _ _ _ _ _ _ _ _ _ w731 _ _ _ _ _ _ _ _ _ _ _ _ _ _ _ _ _ _ _ _ _ _ _ _ _ _ _] -> w689
              tunnel: [_ _ _ _ _ _ _ _ _ _ _ _ _ _ _ _ _ _ _ _ _ w732 _ _ _ _ _ _ _ _ _ _ _ _ _ _ _ _ _ _ _ _ _ _ _ _ _ _] -> w688
              tunnel: [_ _ _ _ _ _ _ _ _ _ _ _ _ _ _ _ _ _ _ _ _ _ w733 _ _ _ _ _ _ _ _ _ _ _ _ _ _ _ _ _ _ _ _ _ _ _ _ _] -> w686
              tunnel: [_ _ _ _ _ _ _ _ _ _ _ _ _ _ _ _ _ _ _ _ _ _ _ w734 _ _ _ _ _ _ _ _ _ _ _ _ _ _ _ _ _ _ _ _ _ _ _ _] -> w687
              tunnel: [_ _ _ _ _ _ _ _ _ _ _ _ _ _ _ _ _ _ _ _ _ _ _ _ w735 _ _ _ _ _ _ _ _ _ _ _ _ _ _ _ _ _ _ _ _ _ _ _] -> w683
              tunnel: [_ _ _ _ _ _ _ _ _ _ _ _ _ _ _ _ _ _ _ _ _ _ _ _ _ w736 _ _ _ _ _ _ _ _ _ _ _ _ _ _ _ _ _ _ _ _ _ _] -> w682
              tunnel: [_ _ _ _ _ _ _ _ _ _ _ _ _ _ _ _ _ _ _ _ _ _ _ _ _ _ w737 _ _ _ _ _ _ _ _ _ _ _ _ _ _ _ _ _ _ _ _ _] -> w681
              tunnel: [_ _ _ _ _ _ _ _ _ _ _ _ _ _ _ _ _ _ _ _ _ _ _ _ _ _ _ w738 _ _ _ _ _ _ _ _ _ _ _ _ _ _ _ _ _ _ _ _] -> w680
              tunnel: [_ _ _ _ _ _ _ _ _ _ _ _ _ _ _ _ _ _ _ _ _ _ _ _ _ _ _ _ w739 _ _ _ _ _ _ _ _ _ _ _ _ _ _ _ _ _ _ _] -> w679
              tunnel: [_ _ _ _ _ _ _ _ _ _ _ _ _ _ _ _ _ _ _ _ _ _ _ _ _ _ _ _ _ w740 _ _ _ _ _ _ _ _ _ _ _ _ _ _ _ _ _ _] -> w678
              tunnel: [_ _ _ _ _ _ _ _ _ _ _ _ _ _ _ _ _ _ _ _ _ _ _ _ _ _ _ _ _ _ w741 _ _ _ _ _ _ _ _ _ _ _ _ _ _ _ _ _] -> w677
              tunnel: [_ _ _ _ _ _ _ _ _ _ _ _ _ _ _ _ _ _ _ _ _ _ _ _ _ _ _ _ _ _ _ w742 _ _ _ _ _ _ _ _ _ _ _ _ _ _ _ _] -> w676
              tunnel: [_ _ _ _ _ _ _ _ _ _ _ _ _ _ _ _ _ _ _ _ _ _ _ _ _ _ _ _ _ _ _ _ w743 _ _ _ _ _ _ _ _ _ _ _ _ _ _ _] -> w675
              tunnel: [_ _ _ _ _ _ _ _ _ _ _ _ _ _ _ _ _ _ _ _ _ _ _ _ _ _ _ _ _ _ _ _ _ w744 _ _ _ _ _ _ _ _ _ _ _ _ _ _] -> w674
              tunnel: [_ _ _ _ _ _ _ _ _ _ _ _ _ _ _ _ _ _ _ _ _ _ _ _ _ _ _ _ _ _ _ _ _ _ w745 _ _ _ _ _ _ _ _ _ _ _ _ _] -> w673
              tunnel: [_ _ _ _ _ _ _ _ _ _ _ _ _ _ _ _ _ _ _ _ _ _ _ _ _ _ _ _ _ _ _ _ _ _ _ w746 _ _ _ _ _ _ _ _ _ _ _ _] -> w672
              tunnel: [_ _ _ _ _ _ _ _ _ _ _ _ _ _ _ _ _ _ _ _ _ _ _ _ _ _ _ _ _ _ _ _ _ _ _ _ w747 _ _ _ _ _ _ _ _ _ _ _] -> w671
              tunnel: [_ _ _ _ _ _ _ _ _ _ _ _ _ _ _ _ _ _ _ _ _ _ _ _ _ _ _ _ _ _ _ _ _ _ _ _ _ w748 _ _ _ _ _ _ _ _ _ _] -> w670
              tunnel: [_ _ _ _ _ _ _ _ _ _ _ _ _ _ _ _ _ _ _ _ _ _ _ _ _ _ _ _ _ _ _ _ _ _ _ _ _ _ w749 _ _ _ _ _ _ _ _ _] -> w669
              tunnel: [_ _ _ _ _ _ _ _ _ _ _ _ _ _ _ _ _ _ _ _ _ _ _ _ _ _ _ _ _ _ _ _ _ _ _ _ _ _ _ w750 _ _ _ _ _ _ _ _] -> w668
              tunnel: [_ _ _ _ _ _ _ _ _ _ _ _ _ _ _ _ _ _ _ _ _ _ _ _ _ _ _ _ _ _ _ _ _ _ _ _ _ _ _ _ w751 _ _ _ _ _ _ _] -> w667
              tunnel: [_ _ _ _ _ _ _ _ _ _ _ _ _ _ _ _ _ _ _ _ _ _ _ _ _ _ _ _ _ _ _ _ _ _ _ _ _ _ _ _ _ w752 _ _ _ _ _ _] -> w666
              tunnel: [_ _ _ _ _ _ _ _ _ _ _ _ _ _ _ _ _ _ _ _ _ _ _ _ _ _ _ _ _ _ _ _ _ _ _ _ _ _ _ _ _ _ w753 _ _ _ _ _] -> w665
              tunnel: [_ _ _ _ _ _ _ _ _ _ _ _ _ _ _ _ _ _ _ _ _ _ _ _ _ _ _ _ _ _ _ _ _ _ _ _ _ _ _ _ _ _ _ w754 _ _ _ _] -> w664
              tunnel: [_ _ _ _ _ _ _ _ _ _ _ _ _ _ _ _ _ _ _ _ _ _ _ _ _ _ _ _ _ _ _ _ _ _ _ _ _ _ _ _ _ _ _ _ w755 _ _ _] -> w663
              tunnel: [_ _ _ _ _ _ _ _ _ _ _ _ _ _ _ _ _ _ _ _ _ _ _ _ _ _ _ _ _ _ _ _ _ _ _ _ _ _ _ _ _ _ _ _ _ w756 _ _] -> w662
              tunnel: [_ _ _ _ _ _ _ _ _ _ _ _ _ _ _ _ _ _ _ _ _ _ _ _ _ _ _ _ _ _ _ _ _ _ _ _ _ _ _ _ _ _ _ _ _ _ w757 _] -> w661
              tunnel: [_ _ _ _ _ _ _ _ _ _ _ _ _ _ _ _ _ _ _ _ _ _ _ _ _ _ _ _ _ _ _ _ _ _ _ _ _ _ _ _ _ _ _ _ _ _ _ w758] -> w660
              frame #0 {
                n483 = property on="P1 Piece" class="Pict"() -> ("Position"=w711:T1)  [unwired: 2 in, 2 out]
              }
              frame #1 {
                n484 = property on="P1 Piece 2" class="Pict"() -> ("Position"=w712:T1)  [unwired: 2 in, 2 out]
              }
              frame #2 {
                n485 = property on="P1 Piece 3" class="Pict"() -> ("Position"=w713:T1)  [unwired: 2 in, 2 out]
              }
              frame #3 {
                n486 = property on="P1 Piece 4" class="Pict"() -> ("Position"=w714:T1)  [unwired: 2 in, 2 out]
              }
              frame #4 {
                n487 = property on="P1 Piece 5" class="Pict"() -> ("Position"=w715:T1)  [unwired: 2 in, 2 out]
              }
              frame #5 {
                n488 = property on="P1 Piece 6" class="Pict"() -> ("Position"=w716:T1)  [unwired: 2 in, 2 out]
              }
              frame #6 {
                n489 = property on="P1 Piece 7" class="Pict"() -> ("Position"=w717:T1)  [unwired: 2 in, 2 out]
              }
              frame #7 {
                n490 = property on="P1 Piece 8" class="Pict"() -> ("Position"=w718:T1)  [unwired: 2 in, 2 out]
              }
              frame #8 {
                n491 = property on="P1 Piece 9" class="Pict"() -> ("Position"=w719:T1)  [unwired: 2 in, 2 out]
              }
              frame #9 {
                n492 = property on="P1 Piece 10" class="Pict"() -> ("Position"=w720:T1)  [unwired: 2 in, 2 out]
              }
              frame #10 {
                n493 = property on="P1 Piece 11" class="Pict"() -> ("Position"=w721:T1)  [unwired: 2 in, 2 out]
              }
              frame #11 {
                n494 = property on="P1 Piece 12" class="Pict"() -> ("Position"=w722:T1)  [unwired: 2 in, 2 out]
              }
              frame #12 {
                n495 = property on="P2 Piece" class="Pict"() -> ("Position"=w723:T1)  [unwired: 2 in, 2 out]
              }
              frame #13 {
                n496 = property on="P2 Piece 2" class="Pict"() -> ("Position"=w724:T1)  [unwired: 2 in, 2 out]
              }
              frame #14 {
                n497 = property on="P2 Piece 3" class="Pict"() -> ("Position"=w725:T1)  [unwired: 2 in, 2 out]
              }
              frame #15 {
                n498 = property on="P2 Piece 4" class="Pict"() -> ("Position"=w726:T1)  [unwired: 2 in, 2 out]
              }
              frame #16 {
                n499 = property on="P2 Piece 5" class="Pict"() -> ("Position"=w727:T1)  [unwired: 2 in, 2 out]
              }
              frame #17 {
                n500 = property on="P2 Piece 6" class="Pict"() -> ("Position"=w728:T1)  [unwired: 2 in, 2 out]
              }
              frame #18 {
                n501 = property on="P2 Piece 7" class="Pict"() -> ("Position"=w729:T1)  [unwired: 2 in, 2 out]
              }
              frame #19 {
                n502 = property on="P2 Piece 8" class="Pict"() -> ("Position"=w730:T1)  [unwired: 2 in, 2 out]
              }
              frame #20 {
                n503 = property on="P2 Piece 9" class="Pict"() -> ("Position"=w731:T1)  [unwired: 2 in, 2 out]
              }
              frame #21 {
                n504 = property on="P2 Piece 10" class="Pict"() -> ("Position"=w732:T1)  [unwired: 2 in, 2 out]
              }
              frame #22 {
                n505 = property on="P2 Piece 11" class="Pict"() -> ("Position"=w733:T1)  [unwired: 2 in, 2 out]
              }
              frame #23 {
                n506 = property on="P2 Piece 12" class="Pict"() -> ("Position"=w734:T1)  [unwired: 2 in, 2 out]
              }
              frame #24 {
                n507 = property on="P1 King" class="Pict"() -> ("Position"=w735:T1)  [unwired: 2 in, 2 out]
              }
              frame #25 {
                n508 = property on="P1 King 2" class="Pict"() -> ("Position"=w736:T1)  [unwired: 2 in, 2 out]
              }
              frame #26 {
                n509 = property on="P1 King 3" class="Pict"() -> ("Position"=w737:T1)  [unwired: 2 in, 2 out]
              }
              frame #27 {
                n510 = property on="P1 King 4" class="Pict"() -> ("Position"=w738:T1)  [unwired: 2 in, 2 out]
              }
              frame #28 {
                n511 = property on="P1 King 5" class="Pict"() -> ("Position"=w739:T1)  [unwired: 2 in, 2 out]
              }
              frame #29 {
                n512 = property on="P1 King 6" class="Pict"() -> ("Position"=w740:T1)  [unwired: 2 in, 2 out]
              }
              frame #30 {
                n513 = property on="P1 King 7" class="Pict"() -> ("Position"=w741:T1)  [unwired: 2 in, 2 out]
              }
              frame #31 {
                n514 = property on="P1 King 8" class="Pict"() -> ("Position"=w742:T1)  [unwired: 2 in, 2 out]
              }
              frame #32 {
                n515 = property on="P1 King 9" class="Pict"() -> ("Position"=w743:T1)  [unwired: 2 in, 2 out]
              }
              frame #33 {
                n516 = property on="P1 King 10" class="Pict"() -> ("Position"=w744:T1)  [unwired: 2 in, 2 out]
              }
              frame #34 {
                n517 = property on="P1 King 11" class="Pict"() -> ("Position"=w745:T1)  [unwired: 2 in, 2 out]
              }
              frame #35 {
                n518 = property on="P1 King 12" class="Pict"() -> ("Position"=w746:T1)  [unwired: 2 in, 2 out]
              }
              frame #36 {
                n519 = property on="P2 King" class="Pict"() -> ("Position"=w747:T1)  [unwired: 2 in, 2 out]
              }
              frame #37 {
                n520 = property on="P2 King 2" class="Pict"() -> ("Position"=w748:T1)  [unwired: 2 in, 2 out]
              }
              frame #38 {
                n521 = property on="P2 King 3" class="Pict"() -> ("Position"=w749:T1)  [unwired: 2 in, 2 out]
              }
              frame #39 {
                n522 = property on="P2 King 4" class="Pict"() -> ("Position"=w750:T1)  [unwired: 2 in, 2 out]
              }
              frame #40 {
                n523 = property on="P2 King 5" class="Pict"() -> ("Position"=w751:T1)  [unwired: 2 in, 2 out]
              }
              frame #41 {
                n524 = property on="P2 King 6" class="Pict"() -> ("Position"=w752:T1)  [unwired: 2 in, 2 out]
              }
              frame #42 {
                n525 = property on="P2 King 7" class="Pict"() -> ("Position"=w753:T1)  [unwired: 2 in, 2 out]
              }
              frame #43 {
                n526 = property on="P2 King 8" class="Pict"() -> ("Position"=w754:T1)  [unwired: 2 in, 2 out]
              }
              frame #44 {
                n527 = property on="P2 King 9" class="Pict"() -> ("Position"=w755:T1)  [unwired: 2 in, 2 out]
              }
              frame #45 {
                n528 = property on="P2 King 10" class="Pict"() -> ("Position"=w756:T1)  [unwired: 2 in, 2 out]
              }
              frame #46 {
                n529 = property on="P2 King 11" class="Pict"() -> ("Position"=w757:T1)  [unwired: 2 in, 2 out]
              }
              frame #47 {
                n530 = property on="P2 King 12" class="Pict"() -> ("Position"=w758:T1)  [unwired: 2 in, 2 out]
              }
            }
            n531 = Build Array(w710, w709, w708, w707, w706, w705, w704, w703, w702, w701, w700, w699) -> (w698:T1[])
            n532 = Build Array (concatenate)(w698, w697, w696, w695, w694, w693, w692, w691, w690, w689, w688, w686, w687) -> (w685:T1[])
            n533 = Build Array (concatenate)(w685, w683, w682, w681, w680, w679, w678, w677, w676, w675, w674, w673, w672) -> (w684:T1[])
            n534 = Build Array (concatenate)(w684, w671, w670, w669, w668, w667, w666, w665, w664, w663, w662, w661, w660) -> ()  [unwired: 1 out]
          }
        }
      }
    }
  }
  n535 = stacked-sequence {
    frame #0 {
      n536 = call "Checkers P1 Turn Drawer.vi"() -> ("new picture"=→"P1 Top Right Marker":picture)  [unwired: 11 in]
      n537 = property on="P1 Top Right Marker" class="Pict"("Position"=T1 {"Left"=666, "Top"=666}) -> ()  [unwired: 2 in, 2 out]
    }
    frame #1 {
      n538 = call "Checkers P1 Turn Drawer.vi"() -> ("new picture"=→"P1 Top Left Marker":picture)  [unwired: 11 in]
      n539 = property on="P1 Top Left Marker" class="Pict"("Position"=T1 {"Left"=666, "Top"=666}) -> ()  [unwired: 2 in, 2 out]
    }
    frame #2 {
      n540 = call "Checkers P1 Turn Drawer.vi"() -> ("new picture"=→"P1 Bottom Left Marker":picture)  [unwired: 11 in]
      n541 = property on="P1 Bottom Left Marker" class="Pict"("Position"=T1 {"Left"=666, "Top"=666}) -> ()  [unwired: 2 in, 2 out]
    }
    frame #3 {
      n542 = call "Checkers P1 Turn Drawer.vi"() -> ("new picture"=→"P1 Bottom Right Marker":picture)  [unwired: 11 in]
      n543 = property on="P1 Bottom Right Marker" class="Pict"("Position"=T1 {"Left"=666, "Top"=666}) -> ()  [unwired: 2 in, 2 out]
    }
    frame #4 {
      n544 = call "Checkers P2 Turn Drawer.vi"() -> ("new picture"=→"P2 Top Left Marker":picture)  [unwired: 11 in]
      n545 = property on="P2 Top Left Marker" class="Pict"("Position"=T1 {"Left"=666, "Top"=666}) -> ()  [unwired: 2 in, 2 out]
    }
    frame #5 {
      n546 = call "Checkers P2 Turn Drawer.vi"() -> ("new picture"=→"P2 Top Right Marker":picture)  [unwired: 11 in]
      n547 = property on="P2 Top Right Marker" class="Pict"("Position"=T1 {"Left"=666, "Top"=666}) -> ()  [unwired: 2 in, 2 out]
    }
    frame #6 {
      n548 = call "Checkers P2 Turn Drawer.vi"() -> ("new picture"=→"P2 Bottom Left Marker":picture)  [unwired: 11 in]
      n549 = property on="P2 Bottom Left Marker" class="Pict"("Position"=T1 {"Left"=666, "Top"=666}) -> ()  [unwired: 2 in, 2 out]
    }
    frame #7 {
      n550 = call "Checkers P2 Turn Drawer.vi"() -> ("new picture"=→"P2 Bottom Right Marker":picture)  [unwired: 11 in]
      n551 = property on="P2 Bottom Right Marker" class="Pict"("Position"=T1 {"Left"=666, "Top"=666}) -> ()  [unwired: 2 in, 2 out]
    }
  }
  n552 = control-ref of="P2 King"() -> (w5:refnum<vi>)
  n553 = property class="Pict"(reference=w5, error in=w3, "Position"=T1 {"Left"=637, "Top"=183}) -> ()  [unwired: 2 out]
  "Player 1 Label" <- "Player 1" ("String 3")
  "Player 2 Label" <- "Player 2" ("String 4")
